vi "RunMeasurement.vi"(0 "NumberOfDigits":i32, 1 "DeviceNr.":T1, 2 "Image Fast Axis":dbl, 3 "Image Slow Axis":dbl, 4 "Number Fast Axis Steps":dbl, 5 "Number of Stackslides":dbl, 6 "ScanOrientation":string, 7 "error in":errorcluster, 8 "StartPointScanner":dbl[](array[numeric]), 9 "Fast Axis":string, 10 "Fast axis delta":dbl[](array[numeric]), 11 "Slow Axis":string, 12 "Number Slow Axis  Steps":dbl, 13 "Slow Axis Delta":dbl[](array[numeric]), 14 "Stack Axis Delta":dbl[](array[numeric]), 15 "kinetic":sgl, 16 "LineOnOff":bool[](array[boolean]), 17 "scan time for 1 line/sec":dbl=200.0 format="%.3g", 19 "Modulation#":i32, 20 "ArrayOfWaves":dbl[][](array[numeric]), 22 "StartPositionMirror":dbl[](array[numeric])) -> (27 "error out":errorcluster)   [LabVIEW 2011]
uses:
  Utilities/controls/ctlSeqFNs_PI_SysNr.ctl
  Camera/lib/atmcd32d.llb/Error Code Enum typedef.ctl
  Variables/SavPath.vi
  Variables/GlobalSetConfigurationPhysikalInstruments.vi
  Variables/ModulationNiveaus.vi
  Variables/IlluminationPatterns.vi
  Variables/GlobalCameraDebugTemperature.vi
  Variables/GlobalGetTimingsFromCamera.vi
  Variables/ccdChipPixels.vi
  Variables/GlobalSetGetConfigureCamera.vi
  Kinetics/vi/RampOrLin.vi
  Variables/GlobalGetMesaurementStatus.vi
  Variables/AxisSteps.vi
  Variables/ScanDirection.vi
  UserInterface/AxisSttepsToGo.vi
  Variables/GlobalSetGetPositionParameters.vi
panel:
  out "Waveform Chart":dbl(graph)
  out "Focal Plane Scanner":dbl[][](graph)
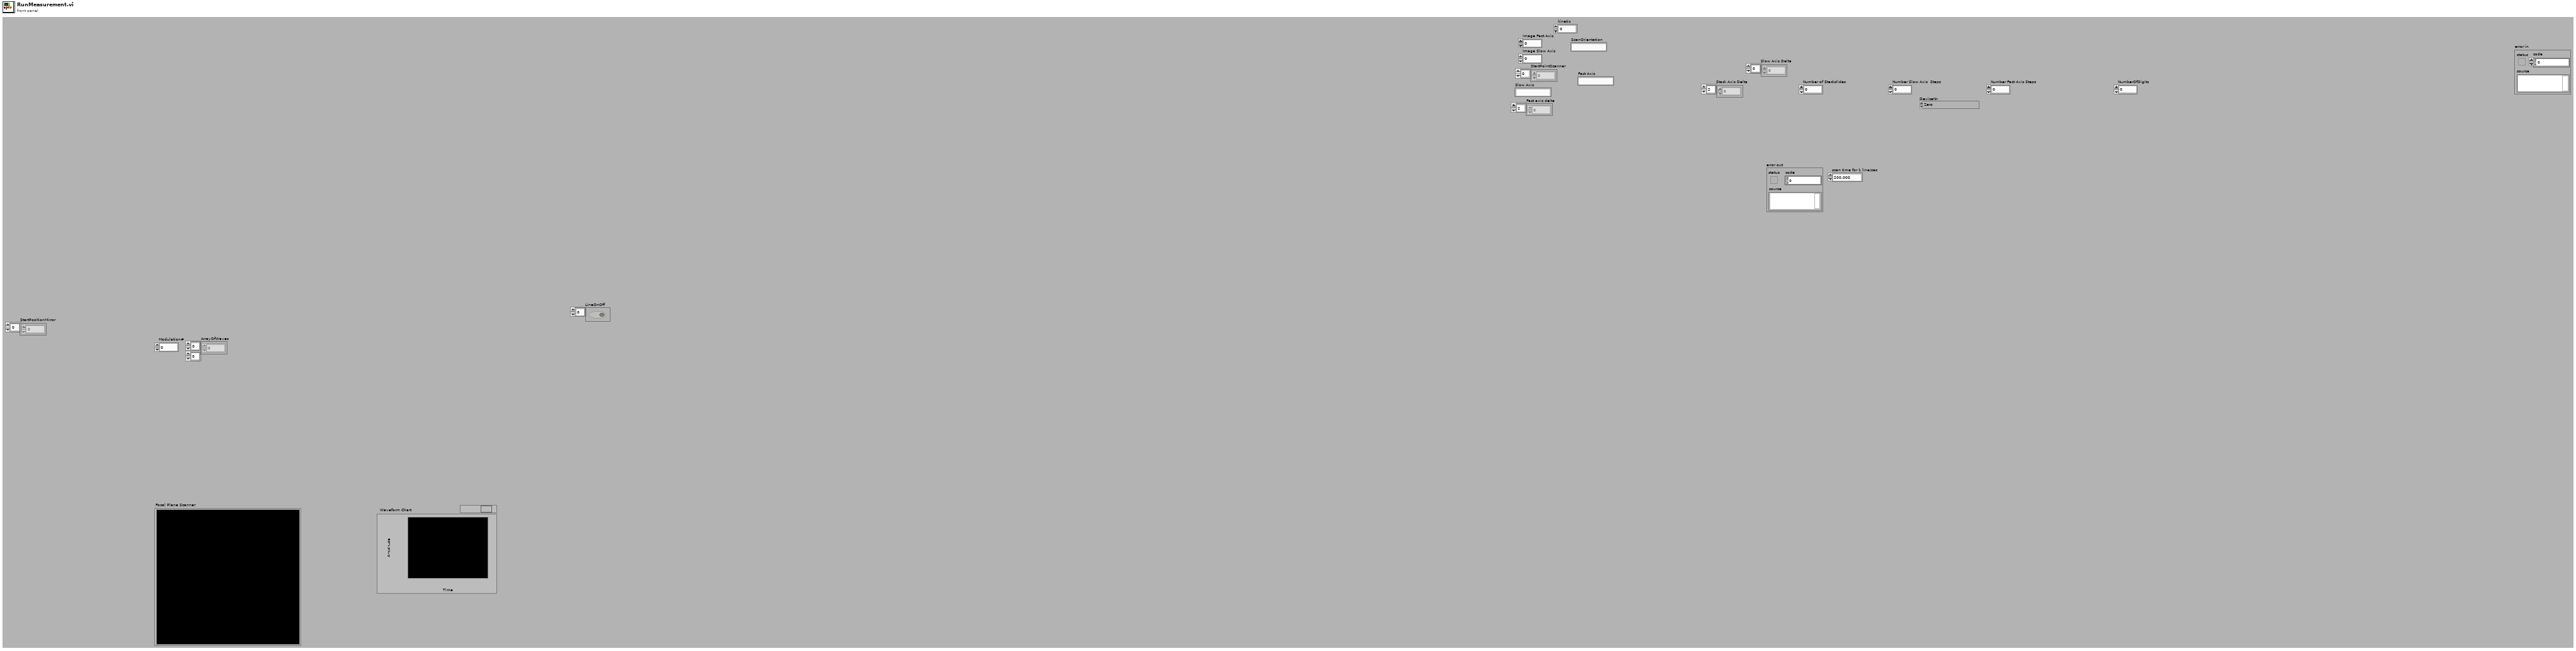
[diagram p1: front panel]
types:
  T1 = typedef "ctlSeqFNs_PI_SysNr.ctl" = enum16{"Zero", "E517", "E710"}
  T2 = typedef "Error Code Enum typedef.ctl" = enum32{"N/A (0)", "DRV_ERROR_CODES", "DRV_SUCCESS", "DRV_VXDNOTINSTALLED", "DRV_ERROR_SCAN", "DRV_ERROR_CHECK_SUM", "DRV_ERROR_FILELOAD", "DRV_UNKNOWN_FUNC", "DRV_ERROR_VXD_INIT", "DRV_ERROR_ADDRESS", "DRV_ERROR_PAGELOCK", "DRV_ERROR_PAGEUNLOCK", "DRV_ERROR_BOARDTEST", "DRV_ERROR_ACK", "DRV_ERROR_UP_FIFO", "DRV_ERROR_PATTERN", "N/A (16)", "DRV_ACQUISITION_ERRORS", "DRV_ACQ_BUFFER", "DRV_ACQ_DOWNFIFO_FULL", "DRV_PROC_UNKONWN_INSTRUCTION", "DRV_ILLEGAL_OP_CODE", "DRV_KINETIC_TIME_NOT_MET", "DRV_ACCUM_TIME_NOT_MET", "DRV_NO_NEW_DATA", "N/A (25)", "DRV_SPOOLERROR", "N/A (27)", "N/A (28)", "N/A (29)", "N/A (30)", "N/A (31)", "N/A (32)", "DRV_TEMPERATURE_CODES", "DRV_TEMPERATURE_OFF", "DRV_TEMPERATURE_NOT_STABILIZED", "DRV_TEMPERATURE_STABILIZED", "DRV_TEMPERATURE_NOT_REACHED", "DRV_TEMPERATURE_OUT_RANGE", "DRV_TEMPERATURE_NOT_SUPPORTED", "DRV_TEMPERATURE_DRIFT", "N/A (41)", "N/A (42)", "N/A (43)", "N/A (44)", "N/A (45)", "N/A (46)", "N/A (47)", "N/A (48)", "DRV_GENERAL_ERRORS", "DRV_INVALID_AUX", "DRV_COF_NOTLOADED", "DRV_FPGAPROG", "DRV_FLEXERROR", "DRV_GPIBERROR", "N/A (55)", "N/A (56)", "N/A (57)", "N/A (58)", "N/A (59)", "N/A (60)", "N/A (61)", "N/A (62)", "N/A (63)", "DRV_DATATYPE", "DRV_DRIVER_ERRORS", "DRV_P1INVALID", "DRV_P2INVALID", "DRV_P3INVALID", "DRV_P4INVALID", "DRV_INIERROR", "DRV_COFERROR", "DRV_ACQUIRING", "DRV_IDLE", "DRV_TEMPCYCLE", "DRV_NOT_INITIALIZED", "DRV_P5INVALID", "DRV_P6INVALID", "DRV_INVALID_MODE", "DRV_INVALID_FILTER", "DRV_I2CERRORS", "DRV_I2CDEVNOTFOUND", "DRV_I2CTIMEOUT", "DRV_P7INVALID", "N/A (84)", "N/A (85)", "N/A (86)", "N/A (87)", "N/A (88)", "N/A (89)", "DRV_IOCERROR", "DRV_VRMVERSIONERROR"}
  T3 = enum32{"Non Linear Illumniation", "Constant Illumination"}
  T4 = cluster{"LineOnOff[0]":bool, "LineOnOff[1]":bool, "LineOnOff[2]":bool, "LineOnOff[3]":bool, "LineOnOff[4]":bool, "LineOnOff[5]":bool, "LineOnOff[6]":bool, "LineOnOff[7]":bool, "LineOnOff[8]":bool}
  T5 = enum16{"open", "replace", "create", "open or create", "replace or create", "replace or create with confirmation"}
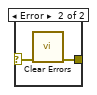
[diagram p2: hidden frame]
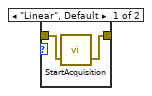
[diagram p3: hidden frame]
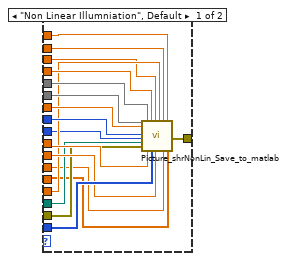
[diagram p6: hidden frame]
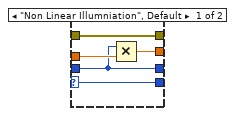
[diagram p7: hidden frame]
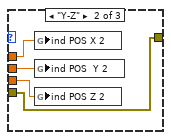
[diagram p9: hidden frame]
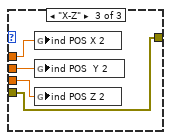
[diagram p10: hidden frame]
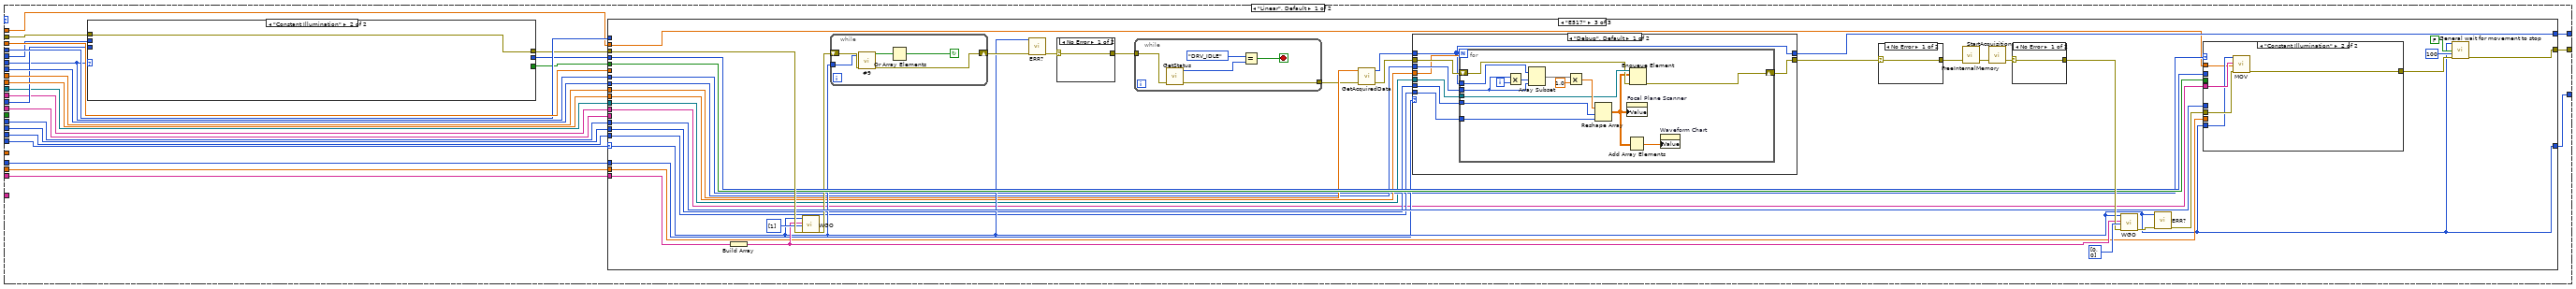
[diagram p11: hidden frame]
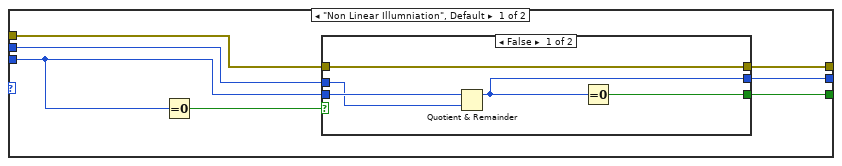
[diagram p12: hidden frame]
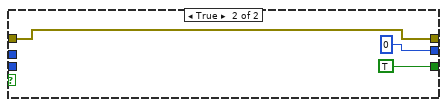
[diagram p13: hidden frame]
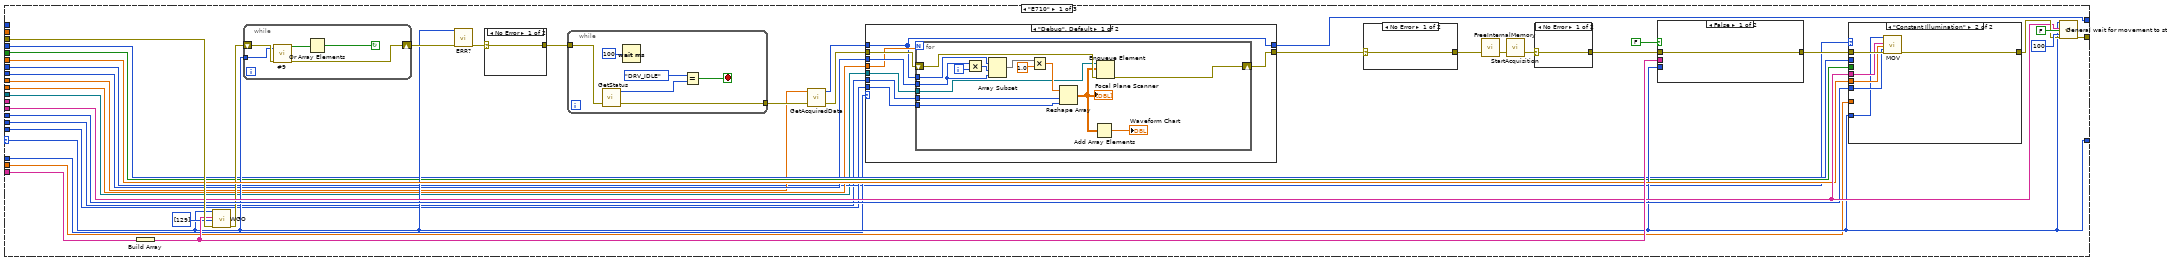
[diagram p14: hidden frame]
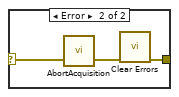
[diagram p16: hidden frame]
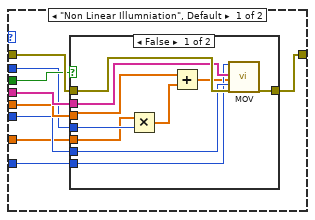
[diagram p17: hidden frame]
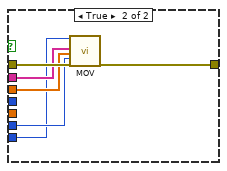
[diagram p18: hidden frame]
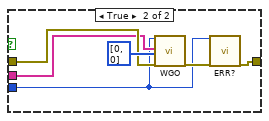
[diagram p19: hidden frame]
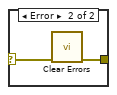
[diagram p20: hidden frame]
diagram:
  n1 = case shown="No Error" "error in" {
    selector: "error in" -> [w66 w113]
    tunnel: ["NumberOfDigits" _] -> w51
    tunnel: [w105 _] -> w50
    tunnel: ["Slow Axis Delta" _] -> w2
    tunnel: ["scan time for 1 line/sec" _] -> _
    tunnel: ["DeviceNr." _] -> w49
    tunnel: ["Stack Axis Delta" _] -> w48
    tunnel: ["Number of Stackslides" _] -> w44
    tunnel: ["Number Slow Axis  Steps" _] -> w43
    tunnel: ["StartPointScanner" _] -> w39
    tunnel: ["Number Fast Axis Steps" _] -> w5
    tunnel: [w89 _] -> w38
    tunnel: [w68 _] -> w37
    tunnel: ["Slow Axis" _] -> w36
    tunnel: ["Fast Axis" _] -> w35
    tunnel: [w56 w113] -> w33
    tunnel: ["Image Slow Axis" _] -> w27
    tunnel: ["ScanOrientation" _] -> w26
    tunnel: [w86 _] -> w25
    tunnel: [w85 _] -> w24
    tunnel: ["Image Fast Axis" _] -> w23
    tunnel: [w83 _] -> w22
    tunnel: [w82 _] -> w21
    tunnel: [w81 _] -> w20
    tunnel: [w80 _] -> w19
    tunnel: ["Fast axis delta" _] -> w18
    tunnel: [w78 _] -> w17
    tunnel: ["kinetic" _] -> w16
    tunnel: [w76 _] -> w14
    tunnel: [w75 _] -> w13
    tunnel: [w72 _] -> w8
    tunnel: ["Modulation#" _] -> w9
    tunnel: ["LineOnOff" _] -> w12
    tunnel: ["ArrayOfWaves" _] -> w7
    tunnel: [w64 _] -> w6
    tunnel: ["StartPositionMirror" _] -> w4
    tunnel: [w61 _] -> w3
    tunnel: [w54 _] -> w1
    frame No Error {
      n2 = call "GetCameraHandle.vi"("error in (no error)"=w66, "cameraIndex"=0) -> ("error out"=w97:errorcluster, "cameraHandle"=w98:i32)  [unwired: 1 in, 1 out]
      n3 = global read "GlobalCameraDebugTemperature.vi" "Fast Slow Debug"() -> (w75:enum32{"Normal", "Debug"})
      n4 = global write "GlobalGetMesaurementStatus.vi" "FifoMesaurementTerminatior"(FALSE ("FifoMesaurementTerminatior")) -> ()
      n5 = global read "GlobalSetConfigurationPhysikalInstruments.vi" "Conn. Axes scanner"() -> (w105:string[])
      n6 = global read "GlobalGetTimingsFromCamera.vi" "Exposure Camera 1"() -> (w76:dbl)
      n7 = global read "GlobalSetConfigurationPhysikalInstruments.vi" "Conn. Axes mirrro"() -> (w61:string[])
      n8 = call "SetCurrentCamera.vi"("error in (no error)"=w97, "cameraHandle"=w98) -> ("error out"=w96:errorcluster)  [unwired: 1 out]
      n9 = global read "RampOrLin.vi" "Kinetice chooser"() -> (w68:enum32{"Linear", "Stepwise"})
      n10 = global read "ccdChipPixels.vi" "CCD Chip Size"() -> (w78:i32)
      n11 = global read "ccdChipPixels.vi" "CCD Chip horizontal start"() -> (w81:i32)
      n12 = global read "ccdChipPixels.vi" "CCD Chip horizontal end"() -> (w80:i32)
      n13 = global read "ccdChipPixels.vi" "CCD Chip Vertical Start"() -> (w82:i32)
      n14 = global read "ccdChipPixels.vi" "CCD Chip Vertical end"() -> (w83:i32)
      n15 = global read "IlluminationPatterns.vi" "Illumination Patterns"() -> (w72:T3)
      n16 = global read "ModulationNiveaus.vi" "ModulationNiveaus"() -> (w64:dbl[])
      n17 = call "GetStatus.vi"("error in (no error)"=w96) -> ("error out"=w91:errorcluster, "status"=w94:T2)  [unwired: 2 in, 1 out]
      n18 = global write "AxisSteps.vi" "Fast_Axis_Steps"("Number Fast Axis Steps") -> ()
      n19 = global write "AxisSteps.vi" "Stack_Steps"("Number of Stackslides") -> ()
      n20 = Not Equal?(x=Error_Code_Enum_typedef."DRV_IDLE" ("status"), y=w94) -> (x != y?=w92:bool)
      n21 = case shown="True" w92 {
        tunnel: w91 -> [w110 w112]
        tunnel: [w110 w111] -> w90
        frame False {
        }
        frame True {
          n22 = call "AbortAcquisition.vi"("error in (no error)"=w112) -> ("error out"=w111:errorcluster)  [unwired: 1 in, 1 out]
        }
      }
      n23 = global write "AxisSteps.vi" "Slow_Axis_Steps"("Number Slow Axis  Steps") -> ()
      n24 = call "FreeInternalMemory.vi"("error in (no error)"=w90) -> ("error out"=w74:errorcluster)  [unwired: 1 in, 1 out]
      n25 = case shown="\"Stepwise\"" w68 {
        tunnel: w74 -> [w108 w109]
        tunnel: [w107 w109] -> w58
        frame "Linear", Default {
          n26 = call "StartAcquisition.vi"("error in (no error)"=w108) -> ("error out"=w107:errorcluster)  [unwired: 1 in, 1 out]
        }
        frame "Stepwise" {
        }
      }
      n27 = Obtain Queue(max queue size (-1, unlimited)=-1, name (unnamed)="PSF", element data type=dbl[][] [], error in (no error)=w58) -> (queue out=w55:refnum<queue>, error out=w57:errorcluster)  [unwired: 1 in, 1 out]
      n28 = Multiply(x=w78, y="Number Fast Axis Steps") -> (x*y=w89:dbl)
      n29 = Flush Queue(queue=w55, error in (no error)=w57) -> (queue out=w54:refnum<queue>, error out=w56:errorcluster)  [unwired: 1 out]
      n30 = global read "GlobalSetGetConfigureCamera.vi" "Hbin"() -> (w86:i32)
      n31 = global read "GlobalSetGetConfigureCamera.vi" "Vbin"() -> (w85:i32)
    }
    frame Error {
    }
  }
  n32 = Subtract(x=w19, y=w20) -> (x-y=w30:i32)
  n33 = Subtract(x=w22, y=w21) -> (x-y=w29:i32)
  n34 = Increment(x=w30) -> (x+1=w11:i32)
  n35 = Increment(x=w29) -> (x+1=w10:i32)
  n36 = for {
    N: w44 -> [_]
    tunnel: w43 -> [w134]
    shift-right: [w140] -> w32
    shift-left: w33 -> [w131]
    tunnel: w50 -> [w152]
    tunnel: w51 -> [w157]
    tunnel: w48 -> [w148]
    tunnel: w35 -> [w162]
    tunnel: w49 -> [w151]
    tunnel: [w141] -> w45 mode=indexing
    tunnel: [w121] -> w46 mode=indexing
    tunnel: [w160] -> w42
    tunnel: [w159] -> w41
    tunnel: [w158] -> w40
    tunnel: w2 -> [w117]
    shift-right: [w143] -> _
    shift-left: w39 -> [w149]
    tunnel: w38 -> [w120]
    tunnel: w37 -> [w128]
    tunnel: w36 -> [w145]
    tunnel: w18 -> [w114]
    tunnel: w5 -> [w135]
    tunnel: w17 -> [w144]
    tunnel: w11 -> [w139]
    tunnel: w10 -> [w138]
    tunnel: w13 -> [w137]
    tunnel: w8 -> [w130]
    tunnel: w9 -> [w125]
    tunnel: w12 -> [w124]
    tunnel: w7 -> [w119]
    shift-right: [w116] -> _
    shift-left: w4 -> [w116]
    tunnel: w3 -> [w118]
    tunnel: w1 -> [w115]
    i -> [w147]
    w142 = ctlSeqFNs_PI_SysNr."E710" ("DeviceNr. 2")
    n37 = Add(x=w149, y=w148) -> (x+y=w143:dbl[])
    n38 = case shown="\"Linear\", Default" w128 {
      selector: w128 -> [w164 w181]
      tunnel: w134 -> [w171 w185]
      tunnel: [w170 w185] -> w133
      tunnel: w125 -> [w169 w184]
      tunnel: [w168 w183] -> w132
      tunnel: w131 -> [w167 w183]
      tunnel: w130 -> [w163 w182]
      tunnel: [w166 w184] -> w129
      tunnel: [w165 w182] -> w127
      tunnel: [w164 w181] -> w126
      frame "Linear", Default {
        n39 = case shown="\"Constant Illumination\"" w163 {
          selector: w163 -> [w172 w177]
          tunnel: w171 -> [w176 w180]
          tunnel: [w175 w180] -> w170
          tunnel: w169 -> [w173 w178]
          tunnel: [w174 w179] -> w168
          tunnel: w167 -> [w174 w179]
          tunnel: [w173 w178] -> w166
          tunnel: [w172 w177] -> w165
          frame "Non Linear Illumniation", Default {
            n40 = Multiply(x=w173, y=w176) -> (x*y=w175:dbl)
          }
          frame "Constant Illumination" {
          }
        }
      }
      frame "Stepwise" {
      }
    }
    n41 = global read "ScanDirection.vi" "ScanDirection"() -> (w146:enum32{"X-Y", "X-Z", "Y-Z", "Focus"})
    n42 = global write "AxisSttepsToGo.vi" "Stack Axis Steps"(w147) -> ()
    n43 = for {
      N: w133 -> [w224]
      shift-right: [w200] -> w123
      shift-left: w132 -> [w236]
      tunnel: w152 -> [w231]
      tunnel: w157 -> [w230]
      tunnel: w162 -> [w237]
      tunnel: w151 -> [w232]
      shift-right: [w207] -> w121
      shift-left: dbl[] [] -> [w208]
      shift-right: [w218] -> w141
      shift-left: dbl[] [] -> [w220]
      tunnel: w117 -> [w235]
      shift-right: [w211] -> _
      shift-left: w143 -> [w228]
      tunnel: w120 -> [w227]
      tunnel: w145 -> [w233]
      tunnel: w114 -> [w229]
      tunnel: w135 -> [w222]
      tunnel: w144 -> [w210]
      tunnel: w139 -> [w225]
      tunnel: w138 -> [w223]
      tunnel: w137 -> [w221]
      tunnel: w129 -> [w216]
      tunnel: w127 -> [w217]
      tunnel: w126 -> [_]
      tunnel: w124 -> [w214]
      tunnel: w128 -> [w212]
      tunnel: w119 -> [w206]
      shift-right: [w205] -> _
      shift-left: w116 -> [w202]
      tunnel: w118 -> [w204]
      tunnel: w117 -> [w203]
      tunnel: w115 -> [w199]
      i -> [w215]
      n44 = Add(x=w203, y=w202) -> (x+y=w205:dbl[])
      n45 = Add(x=w228, y=w235) -> (x+y=w211:dbl[])
      n46 = case shown="\"Stepwise\"" w212 {
        tunnel: [w263 w537] -> w198
        tunnel: w237 -> [w262 w536]
        tunnel: w236 -> [w244 w518]
        tunnel: w232 -> [w261 w517]
        tunnel: [w260 w535] -> w234
        tunnel: w233 -> [_ w534]
        tunnel: w231 -> [w257 w533]
        tunnel: w230 -> [w256 w532]
        tunnel: w229 -> [w250 w531]
        tunnel: w222 -> [w252 w530]
        tunnel: w211 -> [w259 w514]
        tunnel: w210 -> [w253 w529]
        tunnel: [w255 w527] -> w209
        tunnel: w227 -> [w258 _]
        tunnel: w225 -> [w238 w522]
        tunnel: w224 -> [w254 _]
        tunnel: w223 -> [w243 w525]
        tunnel: w221 -> [w251 w526]
        tunnel: w217 -> [w240 w523]
        tunnel: w216 -> [w247 w528]
        tunnel: w215 -> [w246 _]
        tunnel: w214 -> [_ w524]
        tunnel: w206 -> [_ w521]
        tunnel: w205 -> [w242 w515]
        tunnel: w204 -> [w241 _]
        tunnel: w199 -> [w239 w520]
        frame "Linear", Default {
          n47 = case shown="\"Constant Illumination\"" w240 {
            tunnel: w247 -> [w270 _]
            tunnel: [w269 _] -> w249
            tunnel: w246 -> [w267 _]
            tunnel: [w266 _] -> w248
            tunnel: [w265 w279] -> w245
            tunnel: w244 -> [w264 w279]
            frame "Non Linear Illumniation", Default {
              n48 = Equal To 0?(x=w267) -> (x = 0?=w268:bool)
              n49 = case shown="False" w268 {
                tunnel: w267 -> [w275 _]
                tunnel: w270 -> [w274 _]
                tunnel: [w273 TRUE] -> w269
                tunnel: [w272 0] -> w266
                tunnel: [w271 w276] -> w265
                tunnel: w264 -> [w271 w276]
                frame False {
                  n50 = Quotient & Remainder(x=w275, y=w274) -> (x-y*floor(x/y)=w272:i32)  [unwired: 1 out]
                  n51 = Equal To 0?(x=w272) -> (x = 0?=w273:bool)
                }
                frame True {
                }
              }
            }
            frame "Constant Illumination" {
            }
          }
          n52 = case shown="\"E517\"" w261 {
            selector: w261 -> [w298 w401 w421]
            tunnel: [w305 w402 w431] -> w263
            tunnel: w245 -> [w317 w402 w441]
            tunnel: w262 -> [w316 _ w439]
            tunnel: [w298 w401 w421] -> w260
            tunnel: w259 -> [w304 _ _]
            tunnel: w258 -> [w292 _ w418]
            tunnel: w257 -> [w306 _ _]
            tunnel: w256 -> [w303 _ w428]
            tunnel: [w289 _ w420] -> w255
            tunnel: w238 -> [w281 _ w407]
            tunnel: w254 -> [_ _ _]
            tunnel: w243 -> [w290 _ w416]
            tunnel: w253 -> [w294 _ w417]
            tunnel: w252 -> [w291 _ w419]
            tunnel: w251 -> [w293 _ w415]
            tunnel: w249 -> [w297 _ w426]
            tunnel: w250 -> [w296 _ w425]
            tunnel: w248 -> [w295 _ w424]
            tunnel: w240 -> [w282 _ w405]
            tunnel: w242 -> [_ _ w404]
            tunnel: w241 -> [_ _ w406]
            tunnel: w239 -> [w280 _ w403]
            frame "E710" {
              n53 = Build Array(w316) -> (w311:string[])
              n54 = call "WGO.vi"("System no."=w298, "Affected axes"=w311, "WGO Parameter"=i32[] [129], "error in"=w317) -> ("error out"=w300:errorcluster)  [unwired: 14 in, 1 out]
              n55 = while {
                shift-right: [w385] -> w299
                shift-left: w300 -> [w386]
                tunnel: w298 -> [w384]
                stop <- w383 continue-if-true
                n56 = call "#9.vi"("System no."=w384, "error in"=w386) -> ("WG running?"=w387:bool[], "error out"=w385:errorcluster)  [unwired: 16 in]
                n57 = Or Array Elements(Boolean array=w387) -> (logical OR=w383:bool)
              }
              n58 = call "ERR?.vi"("System no."=w298, "error in"=w299) -> ("error out"=w315:errorcluster)  [unwired: 16 in, 1 out]
              n59 = case shown="No Error" w315 {
                selector: w315 -> [w398 w400]
                tunnel: [w398 w399] -> w314
                frame No Error {
                }
                frame Error {
                  n60 = call <vilib>:"Clear Errors.vi"("error in (no error)"=w400) -> ("error out"=w399:errorcluster)  [unwired: 6 in]
                }
              }
              n61 = while {
                tunnel: w314 -> [w346]
                tunnel: [w349] -> w313
                stop <- w348 stop-if-true
                n62 = call "GetStatus.vi"("error in (no error)"=w346) -> ("error out"=w349:errorcluster, "status"=w350:T2)  [unwired: 2 in, 1 out]
                n63 = Wait (ms)(milliseconds to wait=u32 100) -> ()  [unwired: 1 out]
                n64 = Equal?(x=Error_Code_Enum_typedef."DRV_IDLE" ("status"), y=w350) -> (x = y?=w348:bool)
              }
              n65 = call "GetAcquiredData.vi"("error in (no error)"=w313, "size"=w292) -> ("error out"=w286:errorcluster, "array"=w284:i32[])  [unwired: 1 in, 1 out]
              n66 = case shown="\"Debug\", Default" w293 {
                tunnel: w286 -> [w325 w341]
                tunnel: [w324 w341] -> w285
                tunnel: w284 -> [w319 w340]
                tunnel: w294 -> [w323 _]
                tunnel: w281 -> [w322 _]
                tunnel: w290 -> [w321 _]
                tunnel: [w319 w340] -> w289
                tunnel: w291 -> [w320 _]
                tunnel: w280 -> [w318 _]
                frame "Debug", Default {
                  n67 = for {
                    N: w320 -> [_]
                    shift-right: [w328] -> w324
                    shift-left: w325 -> [w329]
                    tunnel: w319 -> [w334]
                    tunnel: w323 -> [w333]
                    tunnel: w322 -> [w332]
                    tunnel: w321 -> [w331]
                    tunnel: w318 -> [w326]
                    i -> [w337]
                    n68 = Multiply(x=w333, y=w337) -> (x*y=w335:i32)
                    n69 = Array Subset(array=w334, index=w335, length=w333) -> (w336:i32[])
                    n70 = Multiply(x=w336, y=1.0) -> (x*y=w339:dbl[])
                    n71 = Reshape Array(w339, w332, w331) -> (w327:dbl[][])
                    "Focal Plane Scanner" <- w327
                    n72 = Add Array Elements(numeric array=w327) -> (sum=→"Waveform Chart":dbl)
                    n73 = Enqueue Element(queue=w326, element=w327, error in (no error)=w329) -> (error out=w328:errorcluster)  [unwired: 1 in, 2 out]
                  }
                }
                frame "Normal" {
                }
              }
              n74 = case shown="No Error" w285 {
                selector: w285 -> [w342 w343]
                tunnel: [w342 w345] -> w287
                frame No Error {
                }
                frame Error {
                  n75 = call "AbortAcquisition.vi"("error in (no error)"=w343) -> ("error out"=w344:errorcluster)  [unwired: 1 in, 1 out]
                  n76 = call <vilib>:"Clear Errors.vi"("error in (no error)"=w344) -> ("error out"=w345:errorcluster)  [unwired: 6 in]
                }
              }
              n77 = call "FreeInternalMemory.vi"("error in (no error)"=w287) -> ("error out"=w283:errorcluster)  [unwired: 1 in, 1 out]
              n78 = call "StartAcquisition.vi"("error in (no error)"=w283) -> ("error out"=w288:errorcluster)  [unwired: 1 in, 1 out]
              n79 = case shown="No Error" w288 {
                selector: w288 -> [w395 w397]
                tunnel: [w395 w396] -> w312
                frame No Error {
                }
                frame Error {
                  n80 = call <vilib>:"Clear Errors.vi"("error in (no error)"=w397) -> ("error out"=w396:errorcluster)  [unwired: 6 in]
                }
              }
              n81 = case shown="False" FALSE {
                tunnel: w312 -> [w388 w393]
                tunnel: w311 -> [_ w392]
                tunnel: [w388 w391] -> w307
                tunnel: w298 -> [_ w389]
                frame False {
                }
                frame True {
                  n82 = call "WGO.vi"("System no."=w389, "Affected axes"=w392, "WGO Parameter"=i32[] [0, 0], "error in"=w393) -> ("error out"=w390:errorcluster)  [unwired: 14 in, 1 out]
                  n83 = call "ERR?.vi"("System no."=w389, "error in"=w390) -> ("error out"=w391:errorcluster)  [unwired: 16 in, 1 out]
                }
              }
              n84 = case shown="\"Constant Illumination\"" w282 {
                tunnel: [w360 w382] -> w308
                tunnel: w307 -> [w359 w381]
                tunnel: w306 -> [w358 w380]
                tunnel: w304 -> [w357 w379]
                tunnel: w303 -> [w356 w378]
                tunnel: w298 -> [w355 w377]
                tunnel: w297 -> [w354 _]
                tunnel: w296 -> [w353 _]
                tunnel: w295 -> [w352 _]
                frame "Non Linear Illumniation", Default {
                  n85 = case shown="False" w354 {
                    tunnel: [w370 w376] -> w360
                    tunnel: w359 -> [w369 w375]
                    tunnel: w358 -> [w368 w374]
                    tunnel: w357 -> [w365 w373]
                    tunnel: w356 -> [w367 w372]
                    tunnel: w355 -> [w366 w371]
                    tunnel: w353 -> [w362 _]
                    tunnel: w352 -> [w363 _]
                    frame False {
                      n86 = Multiply(x=w362, y=w363) -> (x*y=w361:dbl[])
                      n87 = Add(x=w365, y=w361) -> (x+y=w364:dbl[])
                      n88 = call "MOV.vi"("System no."=w366, "Axes to move"=w368, "Position values"=w364, "No.of digits"=w367, "error in"=w369) -> ("error out"=w370:errorcluster)  [unwired: 14 in]
                    }
                    frame True {
                      n89 = call "MOV.vi"("System no."=w371, "Axes to move"=w374, "Position values"=w373, "No.of digits"=w372, "error in"=w375) -> ("error out"=w376:errorcluster)  [unwired: 14 in]
                    }
                  }
                }
                frame "Constant Illumination" {
                  n90 = call "MOV.vi"("System no."=w377, "Axes to move"=w380, "Position values"=w379, "No.of digits"=w378, "error in"=w381) -> ("error out"=w382:errorcluster)  [unwired: 14 in]
                }
              }
              n91 = call "General wait for movement to stop.vi"("System no."=w298, "Axes to wait for"=w306, "All axes?"=FALSE, "Additional wait time, ms"=u32 100, "error in"=w308) -> ("error out"=w305:errorcluster)  [unwired: 13 in, 1 out]
            }
            frame "Zero" {
            }
            frame "E517" {
              n92 = Build Array(w439) -> (w430:string[])
              n93 = call "WGO.vi"("System no."=w421, "Affected axes"=w430, "WGO Parameter"=i32[] [1], "error in"=w441) -> ("error out"=w422:errorcluster)  [unwired: 14 in, 1 out]
              n94 = while {
                shift-right: [w508] -> w423
                shift-left: w422 -> [w509]
                tunnel: w421 -> [w507]
                stop <- w506 continue-if-true
                n95 = call "#9.vi"("System no."=w507, "error in"=w509) -> ("WG running?"=w510:bool[], "error out"=w508:errorcluster)  [unwired: 16 in]
                n96 = Or Array Elements(Boolean array=w510) -> (logical OR=w506:bool)
              }
              n97 = call "ERR?.vi"("System no."=w421, "error in"=w423) -> ("error out"=w438:errorcluster)  [unwired: 16 in, 1 out]
              n98 = case shown="No Error" w438 {
                selector: w438 -> [w511 w513]
                tunnel: [w511 w512] -> w437
                frame No Error {
                }
                frame Error {
                  n99 = call <vilib>:"Clear Errors.vi"("error in (no error)"=w513) -> ("error out"=w512:errorcluster)  [unwired: 6 in]
                }
              }
              n100 = while {
                tunnel: w437 -> [w497]
                tunnel: [w496] -> w409
                stop <- w495 stop-if-true
                n101 = call "GetStatus.vi"("error in (no error)"=w497) -> ("error out"=w496:errorcluster, "status"=w498:T2)  [unwired: 2 in, 1 out]
                n102 = Equal?(x=Error_Code_Enum_typedef."DRV_IDLE" ("status"), y=w498) -> (x = y?=w495:bool)
              }
              n103 = call "GetAcquiredData.vi"("error in (no error)"=w409, "size"=w418) -> ("error out"=w408:errorcluster, "array"=w410:i32[])  [unwired: 1 in, 1 out]
              n104 = case shown="\"Debug\", Default" w415 {
                tunnel: w408 -> [w478 w494]
                tunnel: [w477 w494] -> w411
                tunnel: w410 -> [w472 w493]
                tunnel: w417 -> [w476 _]
                tunnel: w407 -> [w475 _]
                tunnel: w416 -> [w474 _]
                tunnel: [w472 w493] -> w420
                tunnel: w419 -> [w473 _]
                tunnel: w403 -> [w471 _]
                frame "Debug", Default {
                  n105 = for {
                    N: w473 -> [_]
                    shift-right: [w480] -> w477
                    shift-left: w478 -> [w481]
                    tunnel: w472 -> [w487]
                    tunnel: w476 -> [w486]
                    tunnel: w475 -> [w485]
                    tunnel: w474 -> [w484]
                    tunnel: w471 -> [w482]
                    i -> [w490]
                    n106 = Multiply(x=w486, y=w490) -> (x*y=w488:i32)
                    n107 = Array Subset(array=w487, index=w488, length=w486) -> (w489:i32[])
                    n108 = Multiply(x=w489, y=1.0) -> (x*y=w492:dbl[])
                    n109 = Reshape Array(w492, w485, w484) -> (w479:dbl[][])
                    n110 = property on="Focal Plane Scanner" class="IntGraph (strict)"("Value"=w479) -> ()  [unwired: 2 in, 2 out]
                    n111 = Add Array Elements(numeric array=w479) -> (sum=w483:dbl)
                    n112 = Enqueue Element(queue=w482, element=w479, error in (no error)=w481) -> (error out=w480:errorcluster)  [unwired: 1 in, 2 out]
                    n113 = property on="Waveform Chart" class="WFChart (strict)"("Value"=w483) -> ()  [unwired: 2 in, 2 out]
                  }
                }
                frame "Normal" {
                }
              }
              n114 = case shown="No Error" w411 {
                selector: w411 -> [w503 w505]
                tunnel: [w503 w504] -> w412
                frame No Error {
                }
                frame Error {
                  n115 = call <vilib>:"Clear Errors.vi"("error in (no error)"=w505) -> ("error out"=w504:errorcluster)  [unwired: 6 in]
                }
              }
              n116 = call "FreeInternalMemory.vi"("error in (no error)"=w412) -> ("error out"=w414:errorcluster)  [unwired: 1 in, 1 out]
              n117 = call "StartAcquisition.vi"("error in (no error)"=w414) -> ("error out"=w413:errorcluster)  [unwired: 1 in, 1 out]
              n118 = case shown="No Error" w413 {
                selector: w413 -> [w500 w502]
                tunnel: [w500 w501] -> w432
                frame No Error {
                }
                frame Error {
                  n119 = call <vilib>:"Clear Errors.vi"("error in (no error)"=w502) -> ("error out"=w501:errorcluster)  [unwired: 6 in]
                }
              }
              n120 = call "WGO.vi"("System no."=w421, "Affected axes"=w430, "WGO Parameter"=i32[] [0, 0], "error in"=w432) -> ("error out"=w433:errorcluster)  [unwired: 14 in, 1 out]
              n121 = call "ERR?.vi"("System no."=w421, "error in"=w433) -> ("error out"=w429:errorcluster)  [unwired: 16 in, 1 out]
              n122 = case shown="\"Constant Illumination\"" w405 {
                tunnel: w429 -> [w450 w469]
                tunnel: w428 -> [w449 _]
                tunnel: [w448 w470] -> w427
                tunnel: w426 -> [w447 _]
                tunnel: w425 -> [w446 _]
                tunnel: w424 -> [w445 _]
                tunnel: w421 -> [w444 w467]
                tunnel: w404 -> [w443 w466]
                tunnel: w406 -> [w442 w468]
                frame "Non Linear Illumniation", Default {
                  n123 = case shown="True" w447 {
                    tunnel: [w460 w465] -> w448
                    tunnel: w450 -> [w459 w464]
                    tunnel: w442 -> [w458 w463]
                    tunnel: w443 -> [w456 w462]
                    tunnel: w444 -> [w457 w461]
                    tunnel: w449 -> [w453 _]
                    tunnel: w446 -> [w452 _]
                    tunnel: w445 -> [w451 _]
                    frame False {
                      n124 = Multiply(x=w452, y=w451) -> (x*y=w454:dbl[])
                      n125 = Add(x=w456, y=w454) -> (x+y=w455:dbl[])
                      n126 = call "MOV.vi"("System no."=w457, "Axes to move"=w458, "Position values"=w455, "No.of digits"=w453, "error in"=w459) -> ("error out"=w460:errorcluster)  [unwired: 14 in]
                    }
                    frame True {
                      n127 = call "MOV.vi"("System no."=w461, "Axes to move"=w463, "Position values"=w462, "error in"=w464) -> ("error out"=w465:errorcluster)  [unwired: 15 in]
                    }
                  }
                }
                frame "Constant Illumination" {
                  n128 = call "MOV.vi"("System no."=w467, "Axes to move"=w468, "Position values"=w466, "error in"=w469) -> ("error out"=w470:errorcluster)  [unwired: 15 in]
                }
              }
              n129 = call "General wait for movement to stop.vi"("System no."=w421, "All axes?"=FALSE, "Additional wait time, ms"=u32 100, "error in"=w427) -> ("error out"=w431:errorcluster)  [unwired: 14 in, 1 out]
            }
          }
        }
        frame "Stepwise" {
          n130 = case shown="\"Zero\", Default" w517 {
            tunnel: [w538 w540 w542] -> w519
            tunnel: w518 -> [w538 w540 w542]
            tunnel: [_ w539 w541] -> w516
            tunnel: w515 -> [_ _ w541]
            tunnel: w514 -> [_ w539 _]
            frame "Zero", Default {
            }
            frame "E710" {
            }
            frame "E517" {
            }
          }
          n131 = case shown="\"E710\"" w517 {
            selector: w517 -> [w558 w901 w916]
            tunnel: [w551 w902 w917] -> w537
            tunnel: w519 -> [w562 w902 w912]
            tunnel: w536 -> [_ _ _]
            tunnel: [w557 w901 w916] -> w535
            tunnel: w534 -> [_ _ _]
            tunnel: w533 -> [w556 _ w919]
            tunnel: w532 -> [w559 _ w920]
            tunnel: w531 -> [w560 _ w903]
            tunnel: w530 -> [w554 _ w911]
            tunnel: w516 -> [w561 _ w921]
            tunnel: w529 -> [w546 _ w915]
            tunnel: w528 -> [w555 _ w918]
            tunnel: [w550 _ w910] -> w527
            tunnel: w526 -> [w543 _ w904]
            tunnel: w525 -> [w547 _ w907]
            tunnel: w524 -> [w553 _ w914]
            tunnel: w523 -> [w552 _ w913]
            tunnel: w522 -> [w548 _ w908]
            tunnel: w521 -> [w545 _ w906]
            tunnel: w520 -> [w544 _ w905]
            frame "E710" {
              n132 = for {
                N: w554 -> [_]
                tunnel: w558 -> [w582]
                tunnel: w556 -> [w581]
                tunnel: w559 -> [w579]
                shift-right: [w585] -> w551
                shift-left: w562 -> [w577]
                shift-right: [w580] -> _
                shift-left: w561 -> [w588]
                tunnel: w560 -> [w578]
                tunnel: [w582] -> w557
                tunnel: w555 -> [w573]
                tunnel: w553 -> [w574]
                tunnel: w545 -> [w576]
                tunnel: w552 -> [w572]
                tunnel: w546 -> [w571]
                shift-right: [w569] -> w550
                shift-left: i32[] [] -> [w568]
                tunnel: w548 -> [w567]
                tunnel: w547 -> [w566]
                tunnel: w544 -> [w564]
                tunnel: w543 -> [w563]
                i -> [w570]
                n133 = Add(x=w588, y=w578) -> (x+y=w580:dbl[])
                n134 = case shown="\"Constant Illumination\"" w572 {
                  tunnel: w577 -> [w605 w873]
                  tunnel: w576 -> [w604 _]
                  tunnel: [w603 w860] -> w575
                  tunnel: w574 -> [w602 _]
                  tunnel: w573 -> [w601 _]
                  tunnel: w571 -> [w599 w868]
                  tunnel: w570 -> [w598 w870]
                  tunnel: [w596 w869] -> w569
                  tunnel: w568 -> [w600 w867]
                  tunnel: w567 -> [w595 w865]
                  tunnel: w566 -> [w594 w864]
                  tunnel: w564 -> [w593 w862]
                  tunnel: w563 -> [w592 w859]
                  frame "Non Linear Illumniation", Default {
                    n135 = Increment(x=w598) -> (x+1=w597:i32)
                    n136 = for {
                      N: w601 -> [_]
                      tunnel: w602 -> [w620]
                      shift-right: [w621] -> w603
                      shift-left: w605 -> [w642]
                      tunnel: w604 -> [w631] mode=indexing
                      shift-right: [w638] -> w596
                      shift-left: w600 -> [w639]
                      tunnel: w599 -> [w637]
                      tunnel: w597 -> [w635]
                      tunnel: w595 -> [w633]
                      tunnel: w594 -> [w632]
                      tunnel: w593 -> [w611]
                      tunnel: w592 -> [w606]
                      i -> [w636]
                      n137 = Array To Cluster(array=w620) -> (cluster=w653:T4)
                      n138 = Array To Cluster(array=w620) -> (cluster=w630:T4)
                      n139 = Unbundle By Name(w653) -> ("LineOnOff[0]"=w652:bool, "LineOnOff[1]"=w651:bool, "LineOnOff[2]"=w650:bool, "LineOnOff[3]"=w649:bool, "LineOnOff[4]"=w648:bool, "LineOnOff[5]"=w647:bool, "LineOnOff[6]"=w646:bool, "LineOnOff[7]"=w645:bool)
                      n140 = stacked-sequence {
                        seq-local: [w763 _ _ _ _ _ _ _] -> [_ w775 _ _ _ _ _ _]
                        seq-local: [_ w774 _ _ _ _ _ _] -> [_ _ w787 _ _ _ _ _]
                        seq-local: [_ _ w786 _ _ _ _ _] -> [_ _ _ w799 _ _ _ _]
                        seq-local: [_ _ _ w798 _ _ _ _] -> [_ _ _ _ w811 _ _ _]
                        seq-local: [_ _ _ _ w810 _ _ _] -> [_ _ _ _ _ w823 _ _]
                        seq-local: [_ _ _ _ _ w822 _ _] -> [_ _ _ _ _ _ w835 _]
                        seq-local: [_ _ _ _ _ _ w834 _] -> [_ _ _ _ _ _ _ w847]
                        tunnel: [_ _ _ _ _ _ _ w842] -> w643
                        tunnel: tag "Dev2/ao0" ("physical channels") -> [w762 _ _ _ _ _ _ _]
                        tunnel: tag "Dev2/ao1" ("physical channels") -> [_ w773 _ _ _ _ _ _]
                        tunnel: tag "Dev2/ao2" ("physical channels") -> [_ _ w785 _ _ _ _ _]
                        tunnel: tag "Dev2/ao3" ("physical channels") -> [_ _ _ w797 _ _ _ _]
                        tunnel: tag "Dev2/ao4" ("physical channels") -> [_ _ _ _ w809 _ _ _]
                        tunnel: tag "Dev2/ao5" ("physical channels") -> [_ _ _ _ _ w821 _ _]
                        tunnel: tag "Dev2/ao6" ("physical channels") -> [_ _ _ _ _ _ w833 _]
                        tunnel: tag "Dev2/ao7" ("physical channels") -> [_ _ _ _ _ _ _ w846]
                        tunnel: w652 -> [w761 _ _ _ _ _ _ _]
                        tunnel: w651 -> [_ w772 _ _ _ _ _ _]
                        tunnel: w650 -> [_ _ w784 _ _ _ _ _]
                        tunnel: w649 -> [_ _ _ w796 _ _ _ _]
                        tunnel: w648 -> [_ _ _ _ w808 _ _ _]
                        tunnel: w647 -> [_ _ _ _ _ w820 _ _]
                        tunnel: w646 -> [_ _ _ _ _ _ w832 _]
                        tunnel: w645 -> [_ _ _ _ _ _ _ w845]
                        tunnel: [w760 _ _ _ _ _ _ _] -> w619
                        tunnel: [_ w771 _ _ _ _ _ _] -> w618
                        tunnel: [_ _ w783 _ _ _ _ _] -> w617
                        tunnel: [_ _ _ w795 _ _ _ _] -> w616
                        tunnel: [_ _ _ _ _ w819 _ _] -> w614
                        tunnel: [_ _ _ _ _ _ w831 _] -> w613
                        tunnel: [_ _ _ _ _ _ _ w844] -> w612
                        tunnel: w642 -> [w759 _ _ _ _ _ _ _]
                        tunnel: w631 -> [w758 w770 w782 w794 w807 w818 w830 w843]
                        tunnel: [_ _ _ _ w806 _ _ _] -> w615
                        frame #0 {
                          n141 = case shown="True" w761 {
                            tunnel: [w764 w769] -> w763
                            tunnel: w762 -> [_ w768]
                            tunnel: [_ w767] -> w760
                            tunnel: w759 -> [w764 w766]
                            tunnel: w758 -> [_ w765]
                            frame False {
                            }
                            frame True {
                              n142 = call "ModulatorStepwise.vi"("error in (no error)"=w766, "wave"=w765, "physical channels"=w768) -> ("error out"=w769:errorcluster, "task out"=w767:refnum<k21>)  [unwired: 7 in]
                            }
                          }
                        }
                        frame #1 {
                          n143 = case shown="False" w772 {
                            tunnel: w775 -> [w776 w781]
                            tunnel: [w776 w780] -> w774
                            tunnel: w773 -> [_ w779]
                            tunnel: [_ w778] -> w771
                            tunnel: w770 -> [_ w777]
                            frame False {
                            }
                            frame True {
                              n144 = call "ModulatorStepwise.vi"("error in (no error)"=w781, "wave"=w777, "physical channels"=w779) -> ("error out"=w780:errorcluster, "task out"=w778:refnum<k21>)  [unwired: 7 in]
                            }
                          }
                        }
                        frame #2 {
                          n145 = case shown="False" w784 {
                            tunnel: w787 -> [w788 w793]
                            tunnel: [w788 w792] -> w786
                            tunnel: w785 -> [_ w791]
                            tunnel: [_ w790] -> w783
                            tunnel: w782 -> [_ w789]
                            frame False {
                            }
                            frame True {
                              n146 = call "ModulatorStepwise.vi"("error in (no error)"=w793, "wave"=w789, "physical channels"=w791) -> ("error out"=w792:errorcluster, "task out"=w790:refnum<k21>)  [unwired: 7 in]
                            }
                          }
                        }
                        frame #3 {
                          n147 = case shown="False" w796 {
                            tunnel: w799 -> [w800 w805]
                            tunnel: [w800 w804] -> w798
                            tunnel: w797 -> [_ w803]
                            tunnel: [_ w802] -> w795
                            tunnel: w794 -> [_ w801]
                            frame False {
                            }
                            frame True {
                              n148 = call "ModulatorStepwise.vi"("error in (no error)"=w805, "wave"=w801, "physical channels"=w803) -> ("error out"=w804:errorcluster, "task out"=w802:refnum<k21>)  [unwired: 7 in]
                            }
                          }
                        }
                        frame #4 {
                          n149 = case shown="False" w808 {
                            tunnel: w811 -> [w812 w817]
                            tunnel: [w812 w816] -> w810
                            tunnel: w809 -> [_ w815]
                            tunnel: [_ w814] -> w806
                            tunnel: w807 -> [_ w813]
                            frame False {
                            }
                            frame True {
                              n150 = call "ModulatorStepwise.vi"("error in (no error)"=w817, "wave"=w813, "physical channels"=w815) -> ("error out"=w816:errorcluster, "task out"=w814:refnum<k21>)  [unwired: 7 in]
                            }
                          }
                        }
                        frame #5 {
                          n151 = case shown="False" w820 {
                            tunnel: w823 -> [w824 w829]
                            tunnel: [w824 w828] -> w822
                            tunnel: w821 -> [_ w827]
                            tunnel: [_ w826] -> w819
                            tunnel: w818 -> [_ w825]
                            frame False {
                            }
                            frame True {
                              n152 = call "ModulatorStepwise.vi"("error in (no error)"=w829, "wave"=w825, "physical channels"=w827) -> ("error out"=w828:errorcluster, "task out"=w826:refnum<k21>)  [unwired: 7 in]
                            }
                          }
                        }
                        frame #6 {
                          n153 = case shown="True" w832 {
                            tunnel: w835 -> [w836 w841]
                            tunnel: [w836 w840] -> w834
                            tunnel: w833 -> [_ w839]
                            tunnel: [_ w838] -> w831
                            tunnel: w830 -> [_ w837]
                            frame False {
                            }
                            frame True {
                              n154 = call "ModulatorStepwise.vi"("error in (no error)"=w841, "wave"=w837, "physical channels"=w839) -> ("error out"=w840:errorcluster, "task out"=w838:refnum<k21>)  [unwired: 7 in]
                            }
                          }
                        }
                        frame #7 {
                          n155 = case shown="False" w845 {
                            tunnel: w847 -> [w848 w853]
                            tunnel: [w848 w852] -> w842
                            tunnel: w846 -> [_ w851]
                            tunnel: [_ w850] -> w844
                            tunnel: w843 -> [_ w849]
                            frame False {
                            }
                            frame True {
                              n156 = call "ModulatorStepwise.vi"("error in (no error)"=w853, "wave"=w849, "physical channels"=w851) -> ("error out"=w852:errorcluster, "task out"=w850:refnum<k21>)  [unwired: 7 in]
                            }
                          }
                        }
                      }
                      n157 = call "StartAcquisition.vi"("error in (no error)"=w643) -> ("error out"=w661:errorcluster)  [unwired: 1 in, 1 out]
                      n158 = while {
                        tunnel: w661 -> [w856]
                        tunnel: [w855] -> w640
                        stop <- w854 continue-if-true
                        n159 = call "GetStatus.vi"("error in (no error)"=w856) -> ("error out"=w855:errorcluster, "status"=w857:T2)  [unwired: 2 in, 1 out]
                        n160 = Equal?(x=Error_Code_Enum_typedef."DRV_ACQUIRING" ("status"), y=w857) -> (x = y?=w854:bool)
                      }
                      n161 = call "GetAcquiredData.vi"("error in (no error)"=w640, "size"=w637) -> ("error out"=w608:errorcluster, "array"=w641:i32[])  [unwired: 1 in, 1 out]
                      n162 = Multiply(x=w635, y=w636) -> (x*y=w634:i32)
                      n163 = Insert Into Array(array=w639, index=w634, new element=w641) -> (w638:i32[])
                      n164 = case shown="No Error" w608 {
                        selector: w608 -> [w672 w674]
                        tunnel: [w672 w673] -> w607
                        frame No Error {
                        }
                        frame Error {
                          n165 = call <vilib>:"Clear Errors.vi"("error in (no error)"=w674) -> ("error out"=w673:errorcluster)  [unwired: 6 in]
                        }
                      }
                      n166 = case shown="\"Debug\", Default" w606 {
                        tunnel: w641 -> [w669 _]
                        tunnel: w633 -> [w668 _]
                        tunnel: w632 -> [w667 _]
                        tunnel: w611 -> [w664 _]
                        tunnel: [w663 w671] -> w610
                        tunnel: w607 -> [w662 w671]
                        frame "Debug", Default {
                          n167 = To Double Precision Float(number=w669) -> (double precision float=w670:dbl[])
                          n168 = Reshape Array(w670, w668, w667) -> (w665:dbl[][])
                          n169 = property on="Focal Plane Scanner" class="IntGraph (strict)"("Value"=w665) -> ()  [unwired: 2 in, 2 out]
                          n170 = Add Array Elements(numeric array=w665) -> (sum=w666:dbl)
                          n171 = Enqueue Element(queue=w664, element=w665, error in (no error)=w662) -> (error out=w663:errorcluster)  [unwired: 1 in, 2 out]
                          n172 = property on="Waveform Chart" class="WFChart (strict)"("Value"=w666) -> ()  [unwired: 2 in, 2 out]
                        }
                        frame "Normal" {
                        }
                      }
                      n173 = case shown="No Error" w610 {
                        selector: w610 -> [w675 w677]
                        tunnel: [w675 w676] -> w609
                        frame No Error {
                        }
                        frame Error {
                          n174 = call <vilib>:"Clear Errors.vi"("error in (no error)"=w677) -> ("error out"=w676:errorcluster)  [unwired: 6 in]
                        }
                      }
                      n175 = Unbundle By Name(w630) -> ("LineOnOff[0]"=w629:bool, "LineOnOff[1]"=w627:bool, "LineOnOff[2]"=w626:bool, "LineOnOff[3]"=w625:bool, "LineOnOff[4]"=w624:bool, "LineOnOff[5]"=w623:bool, "LineOnOff[6]"=w622:bool, "LineOnOff[7]"=w628:bool)
                      n176 = stacked-sequence {
                        seq-local: [w678 _ _ _ _ _ _ _] -> [_ w689 _ _ _ _ _ _]
                        seq-local: [_ w688 _ _ _ _ _ _] -> [_ _ w699 _ _ _ _ _]
                        seq-local: [_ _ w698 _ _ _ _ _] -> [_ _ _ w709 _ _ _ _]
                        seq-local: [_ _ _ w708 _ _ _ _] -> [_ _ _ _ w719 _ _ _]
                        seq-local: [_ _ _ _ w718 _ _ _] -> [_ _ _ _ _ w729 _ _]
                        seq-local: [_ _ _ _ _ w728 _ _] -> [_ _ _ _ _ _ w739 _]
                        seq-local: [_ _ _ _ _ _ w738 _] -> [_ _ _ _ _ _ _ w749]
                        tunnel: [_ _ _ _ _ _ _ w748] -> w621
                        tunnel: w609 -> [w681 _ _ _ _ _ _ _]
                        tunnel: w629 -> [w680 _ _ _ _ _ _ _]
                        tunnel: w627 -> [_ w691 _ _ _ _ _ _]
                        tunnel: w626 -> [_ _ w701 _ _ _ _ _]
                        tunnel: w625 -> [_ _ _ w711 _ _ _ _]
                        tunnel: w624 -> [_ _ _ _ w721 _ _ _]
                        tunnel: w623 -> [_ _ _ _ _ w731 _ _]
                        tunnel: w622 -> [_ _ _ _ _ _ w741 _]
                        tunnel: w628 -> [_ _ _ _ _ _ _ w751]
                        tunnel: w619 -> [w679 _ _ _ _ _ _ _]
                        tunnel: w618 -> [_ w690 _ _ _ _ _ _]
                        tunnel: w617 -> [_ _ w700 _ _ _ _ _]
                        tunnel: w616 -> [_ _ _ w710 _ _ _ _]
                        tunnel: w615 -> [_ _ _ _ w720 _ _ _]
                        tunnel: w614 -> [_ _ _ _ _ w730 _ _]
                        tunnel: w613 -> [_ _ _ _ _ _ w740 _]
                        tunnel: w612 -> [_ _ _ _ _ _ _ w750]
                        frame #0 {
                          n177 = case shown="True" w680 {
                            tunnel: [w682 w685] -> w678
                            tunnel: w681 -> [w682 w684]
                            tunnel: w679 -> [_ w683]
                            frame False {
                            }
                            frame True {
                              n178 = call <vilib>:"DAQmx Stop Task.vi"("task/channels in"=w683, "error in"=w684) -> ("task out"=w686:refnum<k21>, "error out"=w687:errorcluster)  [unwired: 12 in]
                              n179 = call <vilib>:"DAQmx Clear Task.vi"("task in"=w686, "error in"=w687) -> ("error out"=w685:errorcluster)  [unwired: 13 in]
                            }
                          }
                        }
                        frame #1 {
                          n180 = case shown="False" w691 {
                            tunnel: [w692 w695] -> w688
                            tunnel: w689 -> [w692 w694]
                            tunnel: w690 -> [_ w693]
                            frame False {
                            }
                            frame True {
                              n181 = call <vilib>:"DAQmx Stop Task.vi"("task/channels in"=w693, "error in"=w694) -> ("task out"=w696:refnum<k21>, "error out"=w697:errorcluster)  [unwired: 12 in]
                              n182 = call <vilib>:"DAQmx Clear Task.vi"("task in"=w696, "error in"=w697) -> ("error out"=w695:errorcluster)  [unwired: 13 in]
                            }
                          }
                        }
                        frame #2 {
                          n183 = case shown="True" w701 {
                            tunnel: [w702 w705] -> w698
                            tunnel: w699 -> [w702 w704]
                            tunnel: w700 -> [_ w703]
                            frame False {
                            }
                            frame True {
                              n184 = call <vilib>:"DAQmx Stop Task.vi"("task/channels in"=w703, "error in"=w704) -> ("task out"=w706:refnum<k21>, "error out"=w707:errorcluster)  [unwired: 12 in]
                              n185 = call <vilib>:"DAQmx Clear Task.vi"("task in"=w706, "error in"=w707) -> ("error out"=w705:errorcluster)  [unwired: 13 in]
                            }
                          }
                        }
                        frame #3 {
                          n186 = case shown="True" w711 {
                            tunnel: [w712 w715] -> w708
                            tunnel: w709 -> [w712 w714]
                            tunnel: w710 -> [_ w713]
                            frame False {
                            }
                            frame True {
                              n187 = call <vilib>:"DAQmx Stop Task.vi"("task/channels in"=w713, "error in"=w714) -> ("task out"=w716:refnum<k21>, "error out"=w717:errorcluster)  [unwired: 12 in]
                              n188 = call <vilib>:"DAQmx Clear Task.vi"("task in"=w716, "error in"=w717) -> ("error out"=w715:errorcluster)  [unwired: 13 in]
                            }
                          }
                        }
                        frame #4 {
                          n189 = case shown="True" w721 {
                            tunnel: [w722 w725] -> w718
                            tunnel: w719 -> [w722 w723]
                            tunnel: w720 -> [_ w724]
                            frame False {
                            }
                            frame True {
                              n190 = call <vilib>:"DAQmx Stop Task.vi"("task/channels in"=w724, "error in"=w723) -> ("task out"=w726:refnum<k21>, "error out"=w727:errorcluster)  [unwired: 12 in]
                              n191 = call <vilib>:"DAQmx Clear Task.vi"("task in"=w726, "error in"=w727) -> ("error out"=w725:errorcluster)  [unwired: 13 in]
                            }
                          }
                        }
                        frame #5 {
                          n192 = case shown="True" w731 {
                            tunnel: [w732 w735] -> w728
                            tunnel: w729 -> [w732 w734]
                            tunnel: w730 -> [_ w733]
                            frame False {
                            }
                            frame True {
                              n193 = call <vilib>:"DAQmx Stop Task.vi"("task/channels in"=w733, "error in"=w734) -> ("task out"=w736:refnum<k21>, "error out"=w737:errorcluster)  [unwired: 12 in]
                              n194 = call <vilib>:"DAQmx Clear Task.vi"("task in"=w736, "error in"=w737) -> ("error out"=w735:errorcluster)  [unwired: 13 in]
                            }
                          }
                        }
                        frame #6 {
                          n195 = case shown="True" w741 {
                            tunnel: [w742 w745] -> w738
                            tunnel: w739 -> [w742 w744]
                            tunnel: w740 -> [_ w743]
                            frame False {
                            }
                            frame True {
                              n196 = call <vilib>:"DAQmx Stop Task.vi"("task/channels in"=w743, "error in"=w744) -> ("task out"=w746:refnum<k21>, "error out"=w747:errorcluster)  [unwired: 12 in]
                              n197 = call <vilib>:"DAQmx Clear Task.vi"("task in"=w746, "error in"=w747) -> ("error out"=w745:errorcluster)  [unwired: 13 in]
                            }
                          }
                        }
                        frame #7 {
                          n198 = case shown="True" w751 {
                            tunnel: [w752 w755] -> w748
                            tunnel: w749 -> [w752 w754]
                            tunnel: w750 -> [_ w753]
                            frame False {
                            }
                            frame True {
                              n199 = call <vilib>:"DAQmx Stop Task.vi"("task/channels in"=w753, "error in"=w754) -> ("task out"=w756:refnum<k21>, "error out"=w757:errorcluster)  [unwired: 12 in]
                              n200 = call <vilib>:"DAQmx Clear Task.vi"("task in"=w756, "error in"=w757) -> ("error out"=w755:errorcluster)  [unwired: 13 in]
                            }
                          }
                        }
                      }
                    }
                  }
                  frame "Constant Illumination" {
                    n201 = call "StartAcquisition.vi"("error in (no error)"=w873) -> ("error out"=w874:errorcluster)  [unwired: 1 in, 1 out]
                    n202 = while {
                      tunnel: w874 -> [w895]
                      tunnel: [w894] -> w871
                      stop <- w893 continue-if-true
                      n203 = call "GetStatus.vi"("error in (no error)"=w895) -> ("error out"=w894:errorcluster, "status"=w896:T2)  [unwired: 2 in, 1 out]
                      n204 = Equal?(x=Error_Code_Enum_typedef."DRV_ACQUIRING" ("status"), y=w896) -> (x = y?=w893:bool)
                    }
                    n205 = call "GetAcquiredData.vi"("error in (no error)"=w871, "size"=w868) -> ("error out"=w866:errorcluster, "array"=w872:i32[])  [unwired: 1 in, 1 out]
                    n206 = case shown="No Error" w866 {
                      selector: w866 -> [w890 w892]
                      tunnel: [w890 w891] -> w863
                      frame No Error {
                      }
                      frame Error {
                        n207 = call <vilib>:"Clear Errors.vi"("error in (no error)"=w892) -> ("error out"=w891:errorcluster)  [unwired: 6 in]
                      }
                    }
                    n208 = Insert Into Array(array=w867, index=w870, new element=w872) -> (w869:i32[])
                    n209 = case shown="\"Debug\", Default" w859 {
                      tunnel: w872 -> [w883 _]
                      tunnel: w865 -> [w882 _]
                      tunnel: w864 -> [w881 _]
                      tunnel: w863 -> [w879 w885]
                      tunnel: [w878 w886] -> _
                      tunnel: w862 -> [w876 w886]
                      tunnel: [w875 w885] -> w861
                      frame "Debug", Default {
                        n210 = To Double Precision Float(number=w883) -> (double precision float=w884:dbl[])
                        n211 = Reshape Array(w884, w882, w881) -> (w877:dbl[][])
                        n212 = Add Array Elements(numeric array=w877) -> (sum=w880:dbl)
                        n213 = property on="Focal Plane Scanner" class="IntGraph (strict)"("Value"=w877) -> ()  [unwired: 2 in, 2 out]
                        n214 = Enqueue Element(queue=w876, element=w877, error in (no error)=w879) -> (queue out=w878:refnum<queue>, error out=w875:errorcluster)  [unwired: 1 in, 1 out]
                        n215 = property on="Waveform Chart" class="WFChart (strict)"("Value"=w880) -> ()  [unwired: 2 in, 2 out]
                      }
                      frame "Normal" {
                      }
                    }
                    n216 = case shown="No Error" w861 {
                      selector: w861 -> [w887 w889]
                      tunnel: [w887 w888] -> w860
                      frame No Error {
                      }
                      frame Error {
                        n217 = call <vilib>:"Clear Errors.vi"("error in (no error)"=w889) -> ("error out"=w888:errorcluster)  [unwired: 6 in]
                      }
                    }
                  }
                }
                n218 = call "MOV.vi"("System no."=w582, "Axes to move"=w581, "Position values"=w580, "No.of digits"=w579, "error in"=w575) -> ("error out"=w583:errorcluster)  [unwired: 14 in]
                n219 = call "General wait for movement to stop.vi"("System no."=w582, "Axes to wait for"=w581, "All axes?"=FALSE, "Additional wait time, ms"=u32 100, "error in"=w583) -> ("error out"=w584:errorcluster)  [unwired: 13 in, 1 out]
                n220 = while {
                  tunnel: w584 -> [w591]
                  tunnel: w582 -> [w590]
                  tunnel: [w589] -> w565
                  stop <- w589 continue-if-true
                  n221 = call "ERR?.vi"("System no."=w590, "error in"=w591) -> ("error out"=w589:errorcluster)  [unwired: 16 in, 1 out]
                }
                n222 = case shown="No Error" w565 {
                  selector: w565 -> [w898 w900]
                  tunnel: [w898 w899] -> w585
                  frame No Error {
                  }
                  frame Error {
                    n223 = call <vilib>:"Clear Errors.vi"("error in (no error)"=w900) -> ("error out"=w899:errorcluster)  [unwired: 6 in]
                  }
                }
              }
            }
            frame "Zero" {
            }
            frame "E517" {
              n224 = for {
                N: w911 -> [_]
                tunnel: w903 -> [w949]
                tunnel: w920 -> [w948]
                tunnel: w919 -> [w947]
                tunnel: w918 -> [w946]
                tunnel: w916 -> [w945]
                tunnel: w911 -> [_]
                tunnel: w915 -> [w926]
                tunnel: w914 -> [w944]
                tunnel: w913 -> [w943]
                shift-right: [w928] -> w917
                shift-left: w912 -> [w934]
                shift-right: [w933] -> _
                shift-left: w921 -> [w950]
                shift-right: [w931] -> w910
                shift-left: i32[] [] -> [w932]
                tunnel: w908 -> [w930]
                tunnel: w907 -> [w929]
                tunnel: w906 -> [w924]
                tunnel: w905 -> [w923]
                tunnel: w904 -> [w922]
                i -> [w927]
                n225 = Add(x=w950, y=w949) -> (x+y=w933:dbl[])
                n226 = case shown="\"Constant Illumination\"" w943 {
                  selector: w943 -> [w964 w1244]
                  tunnel: [w968 w1230] -> w938
                  tunnel: w934 -> [w967 w1243]
                  tunnel: w944 -> [w966 _]
                  tunnel: w946 -> [w965 _]
                  tunnel: [w964 w1244] -> _
                  tunnel: w927 -> [w959 w1240]
                  tunnel: w932 -> [w961 w1239]
                  tunnel: [w960 w1238] -> w931
                  tunnel: w930 -> [w963 w1237]
                  tunnel: w929 -> [w962 w1236]
                  tunnel: w926 -> [w957 w1233]
                  tunnel: w924 -> [w956 _]
                  tunnel: w923 -> [w955 w1231]
                  tunnel: w922 -> [w954 w1226]
                  frame "Non Linear Illumniation", Default {
                    n227 = Increment(x=w959) -> (x+1=w958:i32)
                    n228 = for {
                      N: w965 -> [_]
                      tunnel: w966 -> [w984]
                      shift-right: [w1003] -> w968
                      shift-left: w967 -> [w1006]
                      tunnel: w963 -> [w1002]
                      tunnel: w962 -> [w1001]
                      shift-right: [w999] -> w960
                      shift-left: w961 -> [w1000]
                      tunnel: w958 -> [w996]
                      tunnel: w957 -> [w998]
                      tunnel: w956 -> [w975] mode=indexing
                      tunnel: w955 -> [w974]
                      tunnel: w954 -> [w969]
                      i -> [w997]
                      n229 = Array To Cluster(array=w984) -> (cluster=w1017:T4)
                      n230 = Array To Cluster(array=w984) -> (cluster=w994:T4)
                      n231 = Unbundle By Name(w1017) -> ("LineOnOff[0]"=w1016:bool, "LineOnOff[1]"=w1015:bool, "LineOnOff[2]"=w1014:bool, "LineOnOff[3]"=w1013:bool, "LineOnOff[4]"=w1012:bool, "LineOnOff[5]"=w1011:bool, "LineOnOff[6]"=w1010:bool, "LineOnOff[7]"=w1009:bool)
                      n232 = stacked-sequence {
                        seq-local: [w1130 _ _ _ _ _ _ _] -> [_ w1142 _ _ _ _ _ _]
                        seq-local: [_ w1141 _ _ _ _ _ _] -> [_ _ w1154 _ _ _ _ _]
                        seq-local: [_ _ w1153 _ _ _ _ _] -> [_ _ _ w1166 _ _ _ _]
                        seq-local: [_ _ _ w1165 _ _ _ _] -> [_ _ _ _ w1178 _ _ _]
                        seq-local: [_ _ _ _ w1177 _ _ _] -> [_ _ _ _ _ w1190 _ _]
                        seq-local: [_ _ _ _ _ w1189 _ _] -> [_ _ _ _ _ _ w1202 _]
                        seq-local: [_ _ _ _ _ _ w1201 _] -> [_ _ _ _ _ _ _ w1214]
                        tunnel: [_ _ _ _ _ _ _ w1213] -> w1007
                        tunnel: tag "Dev2/ao0" ("physical channels") -> [w1129 _ _ _ _ _ _ _]
                        tunnel: tag "Dev2/ao1" ("physical channels") -> [_ w1140 _ _ _ _ _ _]
                        tunnel: tag "Dev2/ao2" ("physical channels") -> [_ _ w1152 _ _ _ _ _]
                        tunnel: tag "Dev2/ao3" ("physical channels") -> [_ _ _ w1164 _ _ _ _]
                        tunnel: tag "Dev2/ao4" ("physical channels") -> [_ _ _ _ w1176 _ _ _]
                        tunnel: tag "Dev2/ao5" ("physical channels") -> [_ _ _ _ _ w1188 _ _]
                        tunnel: tag "Dev2/ao6" ("physical channels") -> [_ _ _ _ _ _ w1200 _]
                        tunnel: tag "Dev2/ao7" ("physical channels") -> [_ _ _ _ _ _ _ w1212]
                        tunnel: w1016 -> [w1128 _ _ _ _ _ _ _]
                        tunnel: w1015 -> [_ w1139 _ _ _ _ _ _]
                        tunnel: w1014 -> [_ _ w1151 _ _ _ _ _]
                        tunnel: w1013 -> [_ _ _ w1163 _ _ _ _]
                        tunnel: w1012 -> [_ _ _ _ w1175 _ _ _]
                        tunnel: w1011 -> [_ _ _ _ _ w1187 _ _]
                        tunnel: w1010 -> [_ _ _ _ _ _ w1199 _]
                        tunnel: w1009 -> [_ _ _ _ _ _ _ w1211]
                        tunnel: [w1127 _ _ _ _ _ _ _] -> w983
                        tunnel: [_ w1138 _ _ _ _ _ _] -> w982
                        tunnel: [_ _ w1150 _ _ _ _ _] -> w981
                        tunnel: [_ _ _ w1162 _ _ _ _] -> w980
                        tunnel: [_ _ _ _ w1174 _ _ _] -> w979
                        tunnel: [_ _ _ _ _ w1186 _ _] -> w978
                        tunnel: [_ _ _ _ _ _ w1198 _] -> w977
                        tunnel: [_ _ _ _ _ _ _ w1210] -> w976
                        tunnel: w1006 -> [w1126 _ _ _ _ _ _ _]
                        tunnel: w975 -> [w1125 w1137 w1149 w1161 w1173 w1185 w1197 w1209]
                        frame #0 {
                          n233 = case shown="True" w1128 {
                            tunnel: [w1131 w1136] -> w1130
                            tunnel: w1129 -> [_ w1135]
                            tunnel: [_ w1134] -> w1127
                            tunnel: w1126 -> [w1131 w1133]
                            tunnel: w1125 -> [_ w1132]
                            frame False {
                            }
                            frame True {
                              n234 = call "ModulatorStepwise.vi"("error in (no error)"=w1133, "wave"=w1132, "physical channels"=w1135) -> ("error out"=w1136:errorcluster, "task out"=w1134:refnum<k21>)  [unwired: 7 in]
                            }
                          }
                        }
                        frame #1 {
                          n235 = case shown="True" w1139 {
                            tunnel: w1142 -> [w1143 w1148]
                            tunnel: [w1143 w1147] -> w1141
                            tunnel: w1140 -> [_ w1146]
                            tunnel: [_ w1145] -> w1138
                            tunnel: w1137 -> [_ w1144]
                            frame False {
                            }
                            frame True {
                              n236 = call "ModulatorStepwise.vi"("error in (no error)"=w1148, "wave"=w1144, "physical channels"=w1146) -> ("error out"=w1147:errorcluster, "task out"=w1145:refnum<k21>)  [unwired: 7 in]
                            }
                          }
                        }
                        frame #2 {
                          n237 = case shown="True" w1151 {
                            tunnel: w1154 -> [w1155 w1160]
                            tunnel: [w1155 w1159] -> w1153
                            tunnel: w1152 -> [_ w1158]
                            tunnel: [_ w1157] -> w1150
                            tunnel: w1149 -> [_ w1156]
                            frame False {
                            }
                            frame True {
                              n238 = call "ModulatorStepwise.vi"("error in (no error)"=w1160, "wave"=w1156, "physical channels"=w1158) -> ("error out"=w1159:errorcluster, "task out"=w1157:refnum<k21>)  [unwired: 7 in]
                            }
                          }
                        }
                        frame #3 {
                          n239 = case shown="True" w1163 {
                            tunnel: w1166 -> [w1167 w1172]
                            tunnel: [w1167 w1171] -> w1165
                            tunnel: w1164 -> [_ w1170]
                            tunnel: [_ w1169] -> w1162
                            tunnel: w1161 -> [_ w1168]
                            frame False {
                            }
                            frame True {
                              n240 = call "ModulatorStepwise.vi"("error in (no error)"=w1172, "wave"=w1168, "physical channels"=w1170) -> ("error out"=w1171:errorcluster, "task out"=w1169:refnum<k21>)  [unwired: 7 in]
                            }
                          }
                        }
                        frame #4 {
                          n241 = case shown="True" w1175 {
                            tunnel: w1178 -> [w1179 w1184]
                            tunnel: [w1179 w1183] -> w1177
                            tunnel: w1176 -> [_ w1182]
                            tunnel: [_ w1181] -> w1174
                            tunnel: w1173 -> [_ w1180]
                            frame False {
                            }
                            frame True {
                              n242 = call "ModulatorStepwise.vi"("error in (no error)"=w1184, "wave"=w1180, "physical channels"=w1182) -> ("error out"=w1183:errorcluster, "task out"=w1181:refnum<k21>)  [unwired: 7 in]
                            }
                          }
                        }
                        frame #5 {
                          n243 = case shown="True" w1187 {
                            tunnel: w1190 -> [w1191 w1196]
                            tunnel: [w1191 w1195] -> w1189
                            tunnel: w1188 -> [_ w1194]
                            tunnel: [_ w1193] -> w1186
                            tunnel: w1185 -> [_ w1192]
                            frame False {
                            }
                            frame True {
                              n244 = call "ModulatorStepwise.vi"("error in (no error)"=w1196, "wave"=w1192, "physical channels"=w1194) -> ("error out"=w1195:errorcluster, "task out"=w1193:refnum<k21>)  [unwired: 7 in]
                            }
                          }
                        }
                        frame #6 {
                          n245 = case shown="True" w1199 {
                            tunnel: w1202 -> [w1203 w1208]
                            tunnel: [w1203 w1207] -> w1201
                            tunnel: w1200 -> [_ w1206]
                            tunnel: [_ w1205] -> w1198
                            tunnel: w1197 -> [_ w1204]
                            frame False {
                            }
                            frame True {
                              n246 = call "ModulatorStepwise.vi"("error in (no error)"=w1208, "wave"=w1204, "physical channels"=w1206) -> ("error out"=w1207:errorcluster, "task out"=w1205:refnum<k21>)  [unwired: 7 in]
                            }
                          }
                        }
                        frame #7 {
                          n247 = case shown="True" w1211 {
                            tunnel: w1214 -> [w1215 w1220]
                            tunnel: [w1215 w1219] -> w1213
                            tunnel: w1212 -> [_ w1218]
                            tunnel: [_ w1217] -> w1210
                            tunnel: w1209 -> [_ w1216]
                            frame False {
                            }
                            frame True {
                              n248 = call "ModulatorStepwise.vi"("error in (no error)"=w1220, "wave"=w1216, "physical channels"=w1218) -> ("error out"=w1219:errorcluster, "task out"=w1217:refnum<k21>)  [unwired: 7 in]
                            }
                          }
                        }
                      }
                      n249 = call "StartAcquisition.vi"("error in (no error)"=w1007) -> ("error out"=w1025:errorcluster)  [unwired: 1 in, 1 out]
                      n250 = while {
                        tunnel: w1025 -> [w1223]
                        tunnel: [w1222] -> w1004
                        stop <- w1221 continue-if-true
                        n251 = call "GetStatus.vi"("error in (no error)"=w1223) -> ("error out"=w1222:errorcluster, "status"=w1224:T2)  [unwired: 2 in, 1 out]
                        n252 = Equal?(x=Error_Code_Enum_typedef."DRV_ACQUIRING" ("status"), y=w1224) -> (x = y?=w1221:bool)
                      }
                      n253 = call "GetAcquiredData.vi"("error in (no error)"=w1004, "size"=w998) -> ("error out"=w973:errorcluster, "array"=w1005:i32[])  [unwired: 1 in, 1 out]
                      n254 = Multiply(x=w996, y=w997) -> (x*y=w995:i32)
                      n255 = Insert Into Array(array=w1000, index=w995, new element=w1005) -> (w999:i32[])
                      n256 = case shown="No Error" w973 {
                        selector: w973 -> [w1039 w1041]
                        tunnel: [w1039 w1040] -> w972
                        frame No Error {
                        }
                        frame Error {
                          n257 = call <vilib>:"Clear Errors.vi"("error in (no error)"=w1041) -> ("error out"=w1040:errorcluster)  [unwired: 6 in]
                        }
                      }
                      n258 = case shown="\"Normal\"" w969 {
                        tunnel: w1005 -> [w1033 _]
                        tunnel: w1002 -> [w1032 _]
                        tunnel: w1001 -> [w1031 _]
                        tunnel: w974 -> [w1028 _]
                        tunnel: w972 -> [w1027 w1035]
                        tunnel: [w1026 w1035] -> w971
                        frame "Debug", Default {
                          n259 = To Double Precision Float(number=w1033) -> (double precision float=w1034:dbl[])
                          n260 = Reshape Array(w1034, w1032, w1031) -> (w1029:dbl[][])
                          n261 = property on="Focal Plane Scanner" class="IntGraph (strict)"("Value"=w1029) -> ()  [unwired: 2 in, 2 out]
                          n262 = Add Array Elements(numeric array=w1029) -> (sum=w1030:dbl)
                          n263 = Enqueue Element(queue=w1028, element=w1029, error in (no error)=w1027) -> (error out=w1026:errorcluster)  [unwired: 1 in, 2 out]
                          n264 = property on="Waveform Chart" class="WFChart (strict)"("Value"=w1030) -> ()  [unwired: 2 in, 2 out]
                        }
                        frame "Normal" {
                        }
                      }
                      n265 = case shown="No Error" w971 {
                        selector: w971 -> [w1036 w1038]
                        tunnel: [w1036 w1037] -> w970
                        frame No Error {
                        }
                        frame Error {
                          n266 = call <vilib>:"Clear Errors.vi"("error in (no error)"=w1038) -> ("error out"=w1037:errorcluster)  [unwired: 6 in]
                        }
                      }
                      n267 = Unbundle By Name(w994) -> ("LineOnOff[0]"=w993:bool, "LineOnOff[1]"=w991:bool, "LineOnOff[2]"=w990:bool, "LineOnOff[3]"=w989:bool, "LineOnOff[4]"=w988:bool, "LineOnOff[5]"=w987:bool, "LineOnOff[6]"=w986:bool, "LineOnOff[7]"=w992:bool)
                      n268 = stacked-sequence {
                        seq-local: [w1042 _ _ _ _ _ _ _] -> [_ w1053 _ _ _ _ _ _]
                        seq-local: [_ w1052 _ _ _ _ _ _] -> [_ _ w1063 _ _ _ _ _]
                        seq-local: [_ _ w1062 _ _ _ _ _] -> [_ _ _ w1073 _ _ _ _]
                        seq-local: [_ _ _ w1072 _ _ _ _] -> [_ _ _ _ w1083 _ _ _]
                        seq-local: [_ _ _ _ w1082 _ _ _] -> [_ _ _ _ _ w1093 _ _]
                        seq-local: [_ _ _ _ _ w1092 _ _] -> [_ _ _ _ _ _ w1103 _]
                        seq-local: [_ _ _ _ _ _ w1102 _] -> [_ _ _ _ _ _ _ w1113]
                        tunnel: [_ _ _ _ _ _ _ w1112] -> w985
                        tunnel: w970 -> [w1045 _ _ _ _ _ _ _]
                        tunnel: w993 -> [w1044 _ _ _ _ _ _ _]
                        tunnel: w991 -> [_ w1055 _ _ _ _ _ _]
                        tunnel: w990 -> [_ _ w1065 _ _ _ _ _]
                        tunnel: w989 -> [_ _ _ w1075 _ _ _ _]
                        tunnel: w988 -> [_ _ _ _ w1085 _ _ _]
                        tunnel: w987 -> [_ _ _ _ _ w1095 _ _]
                        tunnel: w986 -> [_ _ _ _ _ _ w1105 _]
                        tunnel: w992 -> [_ _ _ _ _ _ _ w1115]
                        tunnel: w983 -> [w1043 _ _ _ _ _ _ _]
                        tunnel: w982 -> [_ w1054 _ _ _ _ _ _]
                        tunnel: w981 -> [_ _ w1064 _ _ _ _ _]
                        tunnel: w980 -> [_ _ _ w1074 _ _ _ _]
                        tunnel: w979 -> [_ _ _ _ w1084 _ _ _]
                        tunnel: w978 -> [_ _ _ _ _ w1094 _ _]
                        tunnel: w977 -> [_ _ _ _ _ _ w1104 _]
                        tunnel: w976 -> [_ _ _ _ _ _ _ w1114]
                        frame #0 {
                          n269 = case shown="False" w1044 {
                            tunnel: [w1046 w1049] -> w1042
                            tunnel: w1045 -> [w1046 w1048]
                            tunnel: w1043 -> [_ w1047]
                            frame False {
                            }
                            frame True {
                              n270 = call <vilib>:"DAQmx Stop Task.vi"("task/channels in"=w1047, "error in"=w1048) -> ("task out"=w1050:refnum<k21>, "error out"=w1051:errorcluster)  [unwired: 12 in]
                              n271 = call <vilib>:"DAQmx Clear Task.vi"("task in"=w1050, "error in"=w1051) -> ("error out"=w1049:errorcluster)  [unwired: 13 in]
                            }
                          }
                        }
                        frame #1 {
                          n272 = case shown="False" w1055 {
                            tunnel: [w1056 w1059] -> w1052
                            tunnel: w1053 -> [w1056 w1058]
                            tunnel: w1054 -> [_ w1057]
                            frame False {
                            }
                            frame True {
                              n273 = call <vilib>:"DAQmx Stop Task.vi"("task/channels in"=w1057, "error in"=w1058) -> ("task out"=w1060:refnum<k21>, "error out"=w1061:errorcluster)  [unwired: 12 in]
                              n274 = call <vilib>:"DAQmx Clear Task.vi"("task in"=w1060, "error in"=w1061) -> ("error out"=w1059:errorcluster)  [unwired: 13 in]
                            }
                          }
                        }
                        frame #2 {
                          n275 = case shown="False" w1065 {
                            tunnel: [w1066 w1069] -> w1062
                            tunnel: w1063 -> [w1066 w1068]
                            tunnel: w1064 -> [_ w1067]
                            frame False {
                            }
                            frame True {
                              n276 = call <vilib>:"DAQmx Stop Task.vi"("task/channels in"=w1067, "error in"=w1068) -> ("task out"=w1070:refnum<k21>, "error out"=w1071:errorcluster)  [unwired: 12 in]
                              n277 = call <vilib>:"DAQmx Clear Task.vi"("task in"=w1070, "error in"=w1071) -> ("error out"=w1069:errorcluster)  [unwired: 13 in]
                            }
                          }
                        }
                        frame #3 {
                          n278 = case shown="False" w1075 {
                            tunnel: [w1076 w1079] -> w1072
                            tunnel: w1073 -> [w1076 w1078]
                            tunnel: w1074 -> [_ w1077]
                            frame False {
                            }
                            frame True {
                              n279 = call <vilib>:"DAQmx Stop Task.vi"("task/channels in"=w1077, "error in"=w1078) -> ("task out"=w1080:refnum<k21>, "error out"=w1081:errorcluster)  [unwired: 12 in]
                              n280 = call <vilib>:"DAQmx Clear Task.vi"("task in"=w1080, "error in"=w1081) -> ("error out"=w1079:errorcluster)  [unwired: 13 in]
                            }
                          }
                        }
                        frame #4 {
                          n281 = case shown="False" w1085 {
                            tunnel: [w1086 w1089] -> w1082
                            tunnel: w1083 -> [w1086 w1087]
                            tunnel: w1084 -> [_ w1088]
                            frame False {
                            }
                            frame True {
                              n282 = call <vilib>:"DAQmx Stop Task.vi"("task/channels in"=w1088, "error in"=w1087) -> ("task out"=w1090:refnum<k21>, "error out"=w1091:errorcluster)  [unwired: 12 in]
                              n283 = call <vilib>:"DAQmx Clear Task.vi"("task in"=w1090, "error in"=w1091) -> ("error out"=w1089:errorcluster)  [unwired: 13 in]
                            }
                          }
                        }
                        frame #5 {
                          n284 = case shown="True" w1095 {
                            tunnel: [w1096 w1099] -> w1092
                            tunnel: w1093 -> [w1096 w1098]
                            tunnel: w1094 -> [_ w1097]
                            frame False {
                            }
                            frame True {
                              n285 = call <vilib>:"DAQmx Stop Task.vi"("task/channels in"=w1097, "error in"=w1098) -> ("task out"=w1100:refnum<k21>, "error out"=w1101:errorcluster)  [unwired: 12 in]
                              n286 = call <vilib>:"DAQmx Clear Task.vi"("task in"=w1100, "error in"=w1101) -> ("error out"=w1099:errorcluster)  [unwired: 13 in]
                            }
                          }
                        }
                        frame #6 {
                          n287 = case shown="True" w1105 {
                            tunnel: [w1106 w1109] -> w1102
                            tunnel: w1103 -> [w1106 w1108]
                            tunnel: w1104 -> [_ w1107]
                            frame False {
                            }
                            frame True {
                              n288 = call <vilib>:"DAQmx Stop Task.vi"("task/channels in"=w1107, "error in"=w1108) -> ("task out"=w1110:refnum<k21>, "error out"=w1111:errorcluster)  [unwired: 12 in]
                              n289 = call <vilib>:"DAQmx Clear Task.vi"("task in"=w1110, "error in"=w1111) -> ("error out"=w1109:errorcluster)  [unwired: 13 in]
                            }
                          }
                        }
                        frame #7 {
                          n290 = case shown="True" w1115 {
                            tunnel: [w1116 w1119] -> w1112
                            tunnel: w1113 -> [w1116 w1118]
                            tunnel: w1114 -> [_ w1117]
                            frame False {
                            }
                            frame True {
                              n291 = call <vilib>:"DAQmx Stop Task.vi"("task/channels in"=w1117, "error in"=w1118) -> ("task out"=w1120:refnum<k21>, "error out"=w1121:errorcluster)  [unwired: 12 in]
                              n292 = call <vilib>:"DAQmx Clear Task.vi"("task in"=w1120, "error in"=w1121) -> ("error out"=w1119:errorcluster)  [unwired: 13 in]
                            }
                          }
                        }
                      }
                      n293 = case shown="No Error" w985 {
                        selector: w985 -> [w1122 w1124]
                        tunnel: [w1122 w1123] -> w1003
                        frame No Error {
                        }
                        frame Error {
                          n294 = call <vilib>:"Clear Errors.vi"("error in (no error)"=w1124) -> ("error out"=w1123:errorcluster)  [unwired: 6 in]
                        }
                      }
                    }
                  }
                  frame "Constant Illumination" {
                    n295 = call "StartAcquisition.vi"("error in (no error)"=w1243) -> ("error out"=w1242:errorcluster)  [unwired: 1 in, 1 out]
                    n296 = while {
                      tunnel: w1242 -> [w1260]
                      tunnel: [w1259] -> w1241
                      stop <- w1261 continue-if-true
                      n297 = call "GetStatus.vi"("error in (no error)"=w1260) -> ("error out"=w1259:errorcluster, "status"=w1262:T2)  [unwired: 2 in, 1 out]
                      n298 = Equal?(x=Error_Code_Enum_typedef."DRV_ACQUIRING" ("status"), y=w1262) -> (x = y?=w1261:bool)
                    }
                    n299 = call "GetAcquiredData.vi"("error in (no error)"=w1241, "size"=w1233) -> ("error out"=w1234:errorcluster, "array"=w1235:i32[])  [unwired: 1 in, 1 out]
                    n300 = case shown="No Error" w1234 {
                      selector: w1234 -> [w1256 w1258]
                      tunnel: [w1256 w1257] -> w1228
                      frame No Error {
                      }
                      frame Error {
                        n301 = call <vilib>:"Clear Errors.vi"("error in (no error)"=w1258) -> ("error out"=w1257:errorcluster)  [unwired: 6 in]
                      }
                    }
                    n302 = Insert Into Array(array=w1239, index=w1240, new element=w1235) -> (w1238:i32[])
                    n303 = case shown="\"Debug\", Default" w1226 {
                      tunnel: w1237 -> [w1250 _]
                      tunnel: w1236 -> [w1249 _]
                      tunnel: w1235 -> [w1248 _]
                      tunnel: [w1246 _] -> w1232
                      tunnel: [w1245 w1252] -> w1227
                      tunnel: w1228 -> [w1245 w1252]
                      frame "Debug", Default {
                        n304 = To Double Precision Float(number=w1248) -> (double precision float=w1251:dbl[])
                        n305 = Reshape Array(w1251, w1250, w1249) -> (w1246:dbl[][])
                        n306 = Add Array Elements(numeric array=w1246) -> (sum=w1247:dbl)
                        n307 = property on="Focal Plane Scanner" class="IntGraph (strict)"("Value"=w1246) -> ()  [unwired: 2 in, 2 out]
                        n308 = property on="Waveform Chart" class="WFChart (strict)"("Value"=w1247) -> ()  [unwired: 2 in, 2 out]
                      }
                      frame "Normal" {
                      }
                    }
                    n309 = Enqueue Element(queue=w1231, element=w1232, error in (no error)=w1227) -> (error out=w1229:errorcluster)  [unwired: 1 in, 2 out]
                    n310 = case shown="No Error" w1229 {
                      selector: w1229 -> [w1253 w1255]
                      tunnel: [w1253 w1254] -> w1230
                      frame No Error {
                      }
                      frame Error {
                        n311 = call <vilib>:"Clear Errors.vi"("error in (no error)"=w1255) -> ("error out"=w1254:errorcluster)  [unwired: 6 in]
                      }
                    }
                  }
                }
                n312 = Index Array(array=w933) -> (element #1=w937:dbl, element #2=w936:dbl)  [unwired: 2 in]
                n313 = Build Array(w937, w936) -> (w935:dbl[])
                n314 = call "MOV.vi"("System no."=w945, "Axes to move"=w947, "Position values"=w935, "No.of digits"=w948, "error in"=w938) -> ("error out"=w939:errorcluster)  [unwired: 14 in]
                n315 = call "General wait for movement to stop.vi"("System no."=w945, "Axes to wait for"=w947, "All axes?"=FALSE, "Additional wait time, ms"=u32 100, "error in"=w939) -> ("error out"=w940:errorcluster)  [unwired: 13 in, 1 out]
                n316 = while {
                  tunnel: w945 -> [w953]
                  tunnel: w940 -> [w952]
                  tunnel: [w951] -> w925
                  stop <- w951 continue-if-true
                  n317 = call "ERR?.vi"("System no."=w953, "error in"=w952) -> ("error out"=w951:errorcluster)  [unwired: 16 in, 1 out]
                }
                n318 = case shown="No Error" w925 {
                  selector: w925 -> [w1264 w1266]
                  tunnel: [w1264 w1265] -> w928
                  frame No Error {
                  }
                  frame Error {
                    n319 = call <vilib>:"Clear Errors.vi"("error in (no error)"=w1266) -> ("error out"=w1265:errorcluster)  [unwired: 6 in]
                  }
                }
              }
            }
          }
        }
      }
      n320 = global write "AxisSttepsToGo.vi" "Slow Axis Steps"(w215) -> ()
      n321 = To Double Precision Float(number=w209) -> (double precision float=w201:dbl[])
      n322 = call "ERR?.vi"("System no."=w234, "error in"=w198) -> ("error out"=w226:errorcluster)  [unwired: 16 in, 1 out]
      n323 = Build Array (concatenate)(w208, w201) -> (w207:dbl[])
      n324 = case shown="No Error" w226 {
        selector: w226 -> [w1267 w1269]
        tunnel: [w1267 w1268] -> w213
        frame No Error {
        }
        frame Error {
          n325 = call <vilib>:"Clear Errors.vi"("error in (no error)"=w1269) -> ("error out"=w1268:errorcluster)  [unwired: 6 in]
        }
      }
      n326 = call "ExitationIntensityTrace.vi"("error in 2"=w213) -> ("data"=w219:dbl, "error out"=w200:errorcluster)  [unwired: 17 in]
      n327 = Build Array (concatenate)(w220, w219) -> (w218:dbl[])
    }
    n328 = call "MOV.vi"("System no."=w142, "Axes to move"=w152, "Position values"=w143, "No.of digits"=w157, "error in"=w123) -> ("error out"=w153:errorcluster)  [unwired: 14 in]
    n329 = call "General wait for movement to stop.vi"("System no."=w142, "Axes to wait for"=w152, "All axes?"=FALSE, "Additional wait time, ms"=u32 100, "error in"=w153) -> ("error out"=w150:errorcluster)  [unwired: 13 in, 1 out]
    n330 = call "POS?.vi"("System no."=w142, "Axes to query"=w152, "error in"=w150) -> ("Position"=w161:dbl[], "error out"=w156:errorcluster)  [unwired: 15 in]
    n331 = Index Array(array=w161) -> (element #1=w159:dbl, element #2=w158:dbl, element #3=w160:dbl)  [unwired: 3 in]
    n332 = case shown="\"X-Y\", Default" w146 {
      tunnel: [w189 w193 w197] -> w140
      tunnel: w156 -> [w189 w193 w197]
      tunnel: w158 -> [w187 w192 w196]
      tunnel: w159 -> [w188 w191 w195]
      tunnel: w160 -> [w186 w190 w194]
      frame "X-Y", Default {
        n333 = global write "GlobalSetGetPositionParameters.vi" "ind POS X 2"(w188) -> ()
        n334 = global write "GlobalSetGetPositionParameters.vi" "ind POS  Y 2"(w187) -> ()
        n335 = global write "GlobalSetGetPositionParameters.vi" "ind POS Z 2"(w186) -> ()
      }
      frame "Y-Z" {
        n336 = global write "GlobalSetGetPositionParameters.vi" "ind POS X 2"(w191) -> ()
        n337 = global write "GlobalSetGetPositionParameters.vi" "ind POS  Y 2"(w192) -> ()
        n338 = global write "GlobalSetGetPositionParameters.vi" "ind POS Z 2"(w190) -> ()
      }
      frame "X-Z" {
        n339 = global write "GlobalSetGetPositionParameters.vi" "ind POS X 2"(w195) -> ()
        n340 = global write "GlobalSetGetPositionParameters.vi" "ind POS  Y 2"(w196) -> ()
        n341 = global write "GlobalSetGetPositionParameters.vi" "ind POS Z 2"(w194) -> ()
      }
    }
  }
  n342 = Build Array(w11, w10) -> (w28:i32[])
  n343 = case shown="No Error" w32 {
    selector: w32 -> [w1270 w1272]
    tunnel: [w1270 w1271] -> w31
    frame No Error {
    }
    frame Error {
      n344 = call <vilib>:"Clear Errors.vi"("error in (no error)"=w1272) -> ("error out"=w1271:errorcluster)  [unwired: 6 in]
    }
  }
  n345 = global read "SavPath.vi" "SavePath"() -> (w15:path)
  n346 = for {
    tunnel: w26 -> [w1290]
    shift-right: [w1295] -> w47
    shift-left: w31 -> [w1291]
    tunnel: w46 -> [w1308] mode=indexing
    tunnel: w45 -> [w1307] mode=indexing
    tunnel: w16 -> [w1286]
    tunnel: w15 -> [w1285]
    tunnel: w41 -> [w1302]
    tunnel: w5 -> [w1301]
    tunnel: w43 -> [w1293]
    tunnel: w40 -> [w1303]
    tunnel: w42 -> [w1304]
    tunnel: w27 -> [w1299]
    tunnel: w23 -> [w1300]
    tunnel: w25 -> [w1306]
    tunnel: w28 -> [w1305]
    tunnel: w24 -> [w1292]
    tunnel: w14 -> [w1275]
    tunnel: w8 -> [w1274]
    tunnel: w6 -> [w1273]
    i -> [w1310]
    w1276 = "_" ("string")
    n347 = Strip Path(path=w1285) -> (stripped path=w1284:path, name=w1283:string)
    n348 = Increment(x=w1310) -> (x+1=w1309:i32)
    n349 = Path To String(path=w1284) -> (string=w1287:string)
    n350 = Number To Decimal String(number=w1309) -> (decimal integer string=w1280:string)  [unwired: 1 in]
    n351 = Get Date/Time In Seconds() -> (seconds since 1Jan1904=w1279:timestamp)
    n352 = Format Date/Time String(time format string (%c)="%d%m%y_%H%M", seconds (now)=w1279) -> (date/time string=w1277:string)  [unwired: 1 in]
    n353 = Concatenate Strings(w1287, "\\" ("string"), "AreaISM" ("string"), w1276, w1290, w1276, w1280, w1276, w1277, w1276, w1283) -> (w1288:string)
    n354 = String To Path(string=w1288) -> (path=w1289:path)
    n355 = Open/Create/Replace File(file path (use dialog)=w1289, error in=w1291, operation (0:open)=T5."create") -> (refnum out=w1297:refnum<file>, error out=w1296:errorcluster)  [unwired: 4 out]
    n356 = Refnum to Path(1:w1297) -> (0:w1294:path)
    n357 = case shown="\"Constant Illumination\"" w1274 {
      tunnel: w1308 -> [w1328 w1345]
      tunnel: w1307 -> [w1327 w1344]
      tunnel: w1306 -> [w1326 w1343]
      tunnel: w1305 -> [w1325 w1342]
      tunnel: w1304 -> [w1324 w1341]
      tunnel: w1303 -> [w1323 w1340]
      tunnel: w1302 -> [w1322 w1339]
      tunnel: w1301 -> [w1321 w1338]
      tunnel: w1300 -> [w1320 w1337]
      tunnel: w1299 -> [w1319 w1336]
      tunnel: w1296 -> [w1318 w1335]
      tunnel: [w1317 w1334] -> w1295
      tunnel: w1294 -> [w1316 w1333]
      tunnel: w1293 -> [w1315 w1332]
      tunnel: w1292 -> [w1314 w1331]
      tunnel: w1286 -> [w1313 w1330]
      tunnel: w1275 -> [w1312 w1329]
      tunnel: w1273 -> [w1311 _]
      frame "Non Linear Illumniation", Default {
        n358 = call "Picture_shrNonLin_Save_to_matlab.vi"("IntensityDiode"=w1327, "Pos_Y"=w1323, "Horizontal Binning"=w1326, "Vertical Binning"=w1314, 5:"in"=w1316, 6:"in"=w1318, "PSF"=w1328, "Pos_Z"=w1324, "Fast Axis Steps"=w1321, "CCD_Y-X"=w1325, "Exposure Camera"=w1312, "Image Fast Axis"=w1320, "Slow Axis Steps"=w1315, "Image Slow Axis"=w1319, "kinetic"=w1313, "Pos_X"=w1322, "ModulationNiveaus"=w1311) -> ("error out"=w1317:errorcluster)  [unwired: 10 in]
      }
      frame "Constant Illumination" {
        n359 = call "Picture_shr_Save_to_matlab.vi"("IntensityDiode"=w1344, "Pos_Y"=w1340, "Horizontal Binning"=w1343, "Vertical Binning"=w1331, 5:"in"=w1333, 6:"in"=w1335, "PSF"=w1345, "Pos_Z"=w1341, "Fast Axis Steps"=w1338, "CCD_Y-X"=w1342, "Exposure Camera"=w1329, "Image Fast Axis"=w1337, "Slow Axis Steps"=w1332, "Image Slow Axis"=w1336, "kinetic"=w1330, "Pos_X"=w1339) -> ("error out"=w1334:errorcluster)  [unwired: 11 in]
      }
    }
  }
  "error out" <- w47
